vi "CC Main.vi"() -> ()   [LabVIEW 2021]
uses:
  typedefs/CC enum Dither Selection.ctl
  typedefs/CC cluster Hardware Config.ctl
  typedefs/CC cluster Device Index.ctl
  Subsystems/SS cluster Command Queues.ctl
  Subsystems/SS typedef Cmd Queue Reference.ctl
  Subsystems/SS typedef cluster Instrument Command Queue Data.ctl
  hk-channel-class/HK Table/HK Table.lvclass
  typedefs/CC cluster System Settings.ctl
  Subsystems/SS cluster Data Queue type.ctl
  Subsystems/Subsystem Class CryoServer/Subsystem CryoServer.lvclass
  C:/Development/prime/Prime-RIMAS/Subsystems/Subsystem Class.lvclass
  Subsystems/Detector/Detector.lvclass
  Subsystems/Subsystem Class Filter Wheel/Subsystem Filter Wheel.lvclass
  Subsystems/Subsystem Class Telescope/Subsystem Telescope.lvclass
  Subsystems/Subsystem Class Focus/Subsystem Class Focus.lvclass
  Subsystems/Subsystem CryoCooler/Subsystem CryoCooler.lvclass
  Subsystems/Subsystem Pressure Monitor/Subsystem Pressure Monitor.lvclass
  Subsystems/SS cluster Script Status Queue.ctl
  typedefs/CC cluster Observation.ctl
  Observation Queue/CC enum Observation Status.ctl
  Telescope/CC cluster Telescope Offsets.ctl
  typedefs/CC cluster Observation Dither Options.ctl
  library/Activity Log/Activity Log enum Action .ctl
  Subsystems/Subsystem Class.lvclass/Subsystem Class.ctl
  typedefs/CC cluster Script.ctl
  typedefs/CC Script Step.ctl
  typedefs/CC enum Script Action.ctl
  Scripts/CC Rd Wr Script Action.ctl
  typedefs/CC enum Alarm Action.ctl
  Logging/CC enum Current Values Action.ctl
  typedefs/CC cluster Script Status Data.ctl
  Subsystems/SS Read cmd q.vi
  54ac6f3e-f790-48ea-ae38-f3b11f920432.vi
  <vilib>/Utility/TDMS File Viewer/TDMS - File Viewer (NXG Style).vi
  <vilib>/Comparison/Less/Less Functor/Less Functor.lvclass
  <vilib>/regexp/Match Regular Expression.xnode
  Subsystems/Subsystem Class.lvclass
  hk-channel-class/HK Item/HK Item.lvclass
  <vilib>/Utility/TDMS File Viewer/NI_TDMS File Viewer.lvlib
panel:
  in  "Tab Control":T1(tab)
  in  "Priority":i32
  in  "Comment":string
  out "Observation File":string
  in  "Block ID":string
  in  "Images":i32=1 min=1 step=1
  in  "Phase":dbl format="%.1g"
  in  "ROT Offset":dbl
  in  "DECoffset":dbl
  in  "RAoffset":dbl
  in  "Obj Type":string
  in  "Obj Name":string
  in  "Observer":string
  in  "Add to Q top":bool
  in  "Add to Q":bool
  out "Current DEC":string
  out "Current RA":string
  in  "Replace":bool
  in  "Add Obs Row":bool
  in  "Generate Script":bool
  in  "Save Obs List":bool
  in  "Load Obs List":bool
  in  "Radius":dbl format="%.1g"
  in  "Int Time":dbl format="%.1g"
  in  "Spots":i32=1 min=1 step=1
  in  "Dither":T2
  in  "Filter 2":u16(ring) items=["Y", "H", "Open", "J"]
  in  "Filter 1":u16(ring) items=["Z", "Open", "Dark", "NB"]
  in  "DEC":string
  in  "RA":string
  in  "Observation List":i32[](listbox)
  in  "Edit FITS Hdr":bool
  in  "Log 2":bool caption="Log"
  in  "Log":bool
  in  "Export Cryo Data":bool
  out "XY Graph":cluster{timestamp[], dbl[]}[](graph)
  in  "Plot":bool
  in  "Channels":i32[](listbox)
  in  "Open Log":bool
  in  "Note for Log":string
  in  "Send":bool
  in  "Close":bool
  in  "Recent Images":i32(listbox)
  out "Status":string
  out "Progress":u8(slide) scale=0.0..100.0
  out "Current File":string
  in  "Data Folder":path
  out "Temp":bool
  out "Cryo Alarm":bool
  out "Pressure Alarm":bool
  out "Telescope Alarm":bool
  out "FW Alarm":bool
  out "Detector Alarm":bool
  out "Alarm Message":string
  out "Alarm Status":bool
  out "Thumbnail":sgl[][](graph)
  out "Zoom":sgl[][](graph)
  out "Console":string
  out "Waveform Graph":cluster{"image":sgl[]}[](graph)
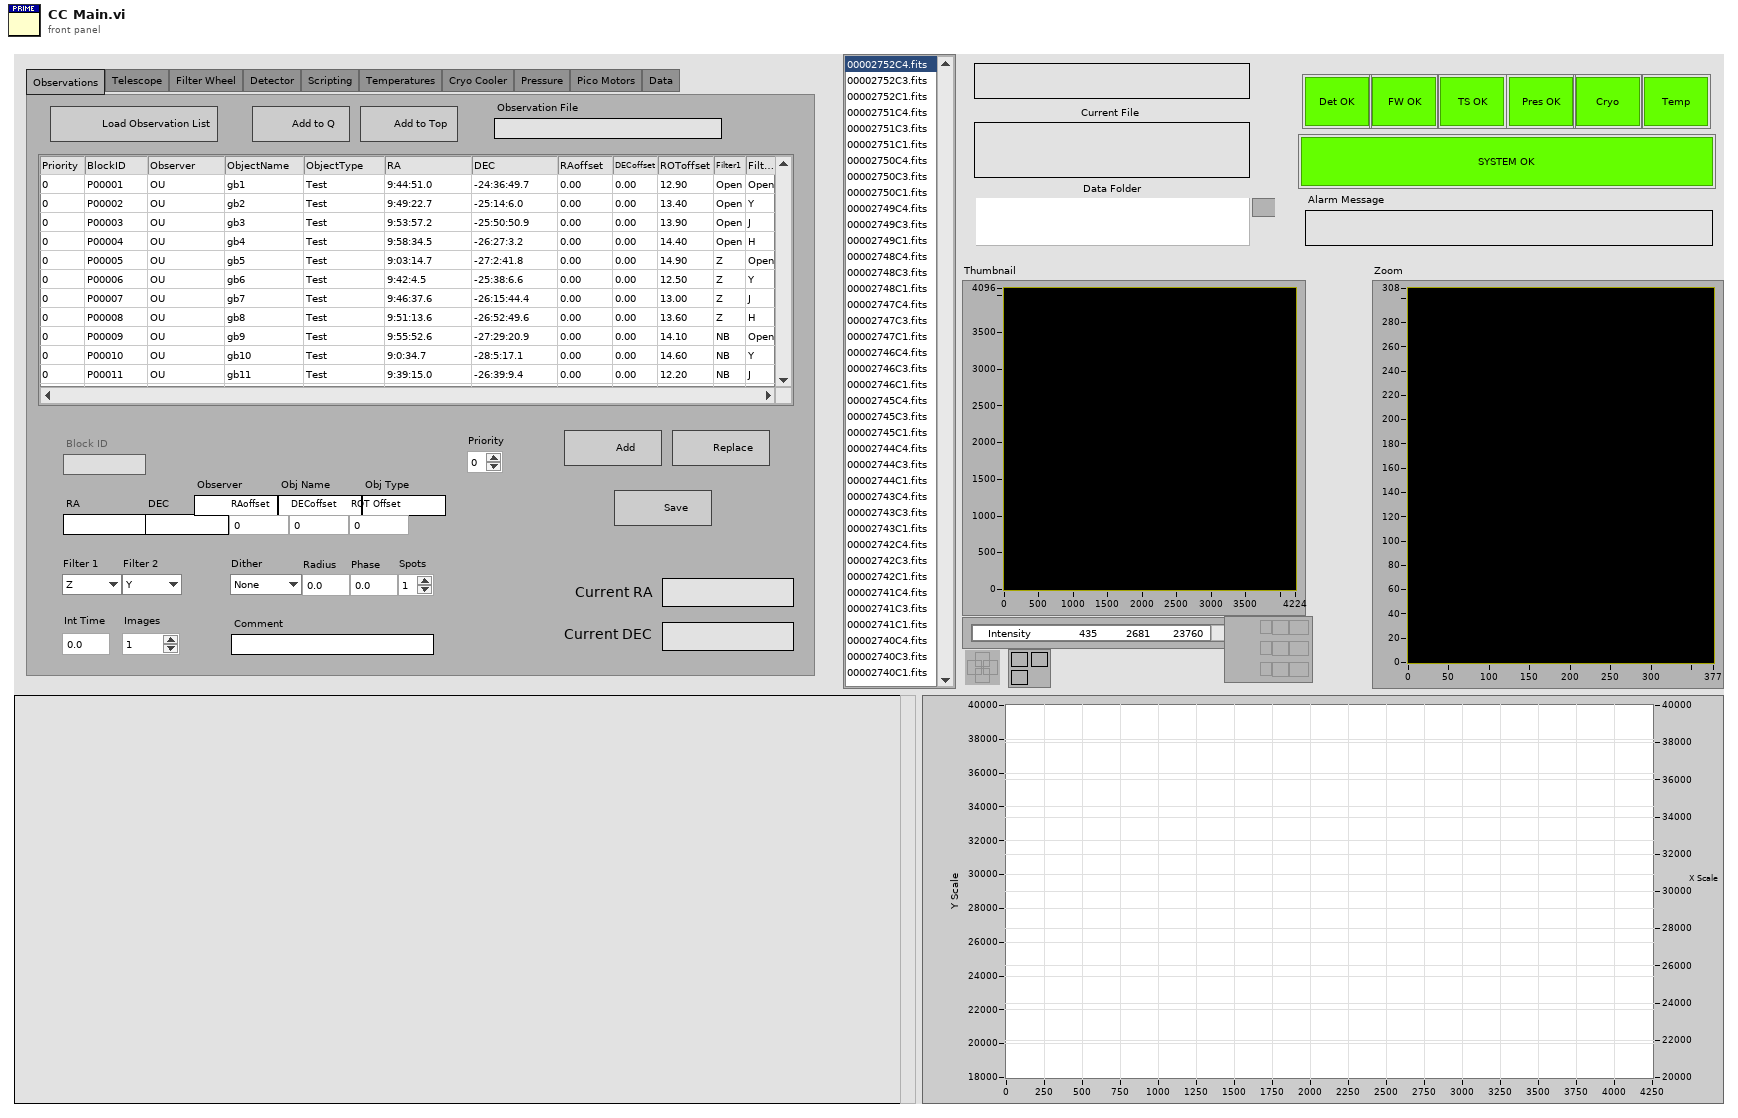
[diagram p1: front panel]
types:
  T1 = enum32{"Observations", "Telescope", "Filter Wheel", "Detector", "Scripting", "Temperatures", "Cryo Cooler", "Pressure", "Pico Motors", "Data"}
  T2 = typedef "CC enum Dither Selection.ctl" = enum16{"None", "Circle", "Random"}
  T3 = enum32{"invalid app kind", "Development System", "Run Time System", "Student Edition", "Embedded LabVIEW", "Evaluation", "Custom"}
  T4 = typedef "CC cluster Hardware Config.ctl" = cluster{"Installed Hardware":T5[]}
  T5 = typedef "CC cluster Device Index.ctl" = cluster{"Device Type Name":string, "Curr Device Name":string, "All Instances":string[]}
  T6 = typedef "SS cluster Command Queues.ctl" = cluster{"Telescope Q":T7, "Filter Wheel Q":T7, "Script Q":T7, "CryoServer Q":T7, "Detector Q":T7, "Focus Q":T7}
  T7 = typedef "SS typedef Cmd Queue Reference.ctl" = refnum<queue>
  T8 = typedef "CC cluster System Settings.ctl" = cluster{"HK Table Name":string, "Images Folder":path, "Obs File":path}
  T9 = typedef "CC cluster Observation.ctl" = cluster{"Priority":i32, "ID":string, "Observer":string, "Obj Name":string, "Obj Type":string, "RA and DEC String":cluster{"RA":string, "DEC":string}, "Filter Wheel 1":string, "Filter Wheel 2":string, "Integration Time":dbl, "Observation Status":T10, "Offsets":T11, "Images":i32, "Dither Options":T12, "Comment 1":string, "Comment 2":string}
  T10 = typedef "CC enum Observation Status.ctl" = enum16{"Ready", "Running", "Done", "Error"}
  T11 = typedef "CC cluster Telescope Offsets.ctl" = cluster{"RA":dbl, "DEC":dbl, "ROT":dbl}
  T12 = typedef "CC cluster Observation Dither Options.ctl" = cluster{"Dither":T2, "Dither Radius":dbl, "Dither Points":i32, "Dither Phase":dbl}
  T13 = cluster{"state":refnum<user-event>, "Hardware":T4, "error":errorcluster, "Cmd Qs":T6, "HK Channels":refnum<class "HK Table.lvclass">, "System Settings":T8, "Data Q":refnum<queue>, "file path":path, "SS":cluster{"CryoServer":refnum<class "Subsystem CryoServer.lvclass">, "Detector":refnum<class "Detector.lvclass">, "Filter Wheel":refnum<class "Subsystem Filter Wheel.lvclass">, "Telescope":refnum<class "Subsystem Telescope.lvclass">, "Focus":refnum<class "Subsystem Class Focus.lvclass">, "CryoCooler":refnum<class "Subsystem CryoCooler.lvclass">, "Pressure":refnum<class "Subsystem Pressure Monitor.lvclass">}, "Script Status Q":refnum<queue>, "Status Data":variant, "curr image":path, "image":sgl[][], "Application:Kind":enum32{"invalid app kind", "Development System", "Run Time System", "Student Edition", "Embedded LabVIEW", "Evaluation", "Custom"}, "Observation List":T9[], "Viewer Ref":refnum<vi>, "Quad Viewer Ref":refnum<vi>, "Obs Queue":refnum<queue>, "Queue vi ref":refnum<vi>, "Script Running":bool}
  T14 = typedef "SS cluster Data Queue type.ctl" = cluster{"Source":string, "Type":string, "Data":variant}
  T15 = typedef "Activity Log enum Action .ctl" = enum16{"Add Entry", "Get Log", "Restore From Disk", "Save to Disk", "Init"}
  T16 = typedef "SS typedef cluster Instrument Command Queue Data.ctl" = cluster{"Cmd":string, "Parameters":variant}
  T17 = typedef "CC Rd Wr Script Action.ctl" = enum16{"Read", "Write", "List", "Delete"}
  T18 = typedef "CC cluster Script.ctl" = cluster{"Name":string, "Script":T19[]}
  T19 = typedef "CC Script Step.ctl" = cluster{"Action":T20, "Data":variant}
  T20 = typedef "CC enum Script Action.ctl" = enum16{"Noop", "Define Object", "Define Exposure", "Define Dithering", "Acquire Images", "Set Filter Wheel", "Telescope Home", "Telescope Move", "Telescope RA DEC", "Focus Move Relative", "Focus Move Absolute", "Focus Set Home", "Macro", "Pause", "Ask User", "Define Random Dither"}
  T21 = typedef "CC enum Alarm Action.ctl" = enum16{"Init", "Add Alarm", "Get Alarms", "Clear Alarm", "Clear All Alarms"}
  T22 = typedef "CC enum Current Values Action.ctl" = enum16{"Init", "Write Item", "Write Array", "Read Item", "Read Array", "Read All", "Add Channels", "New File", "Add Message", "Get Current Values", "Close"}
  T23 = typedef "CC cluster Script Status Data.ctl" = cluster{"Time":timestamp, "Running":bool, "Step":i32, "Script Name":string, "Step Name":string}
  T24 = typedef "SS cluster Script Status Queue.ctl" = cluster{"Msg":string, "Data":variant}
  T25 = enum8{"Enabled", "Disabled", "Disabled and Grayed Out"}
  T26 = typedef "CC cluster Script Panel Defaults.ctl" = cluster{"Script Name":string, "Script Path":path}
  T27 = typedef "CC cluster Alarm Data.ctl" = cluster{"Measured Value":dbl, "Alarm Low":dbl, "Alarm High":dbl, "Message":string, "Source":string}
  T28 = typedef "LVRectTypeDef.ctl" = cluster{"Left":i16, "Top":i16, "Right":i16, "Bottom":i16}
  T29 = cluster{"CryoServer":refnum<class "Subsystem CryoServer.lvclass">, "Detector":refnum<class "Detector.lvclass">, "Filter Wheel":refnum<class "Subsystem Filter Wheel.lvclass">, "Telescope":refnum<class "Subsystem Telescope.lvclass">, "Focus":refnum<class "Subsystem Class Focus.lvclass">, "CryoCooler":refnum<class "Subsystem CryoCooler.lvclass">, "Pressure":refnum<class "Subsystem Pressure Monitor.lvclass">}
  T30 = typedef "LVPoint32TypeDef.ctl" = cluster{"Horizontal":i32, "Vertical":i32}
  T31 = typedef "LVRowAndColumnTypeDef.ctl" = cluster{"Row":i32, "Column":i32}
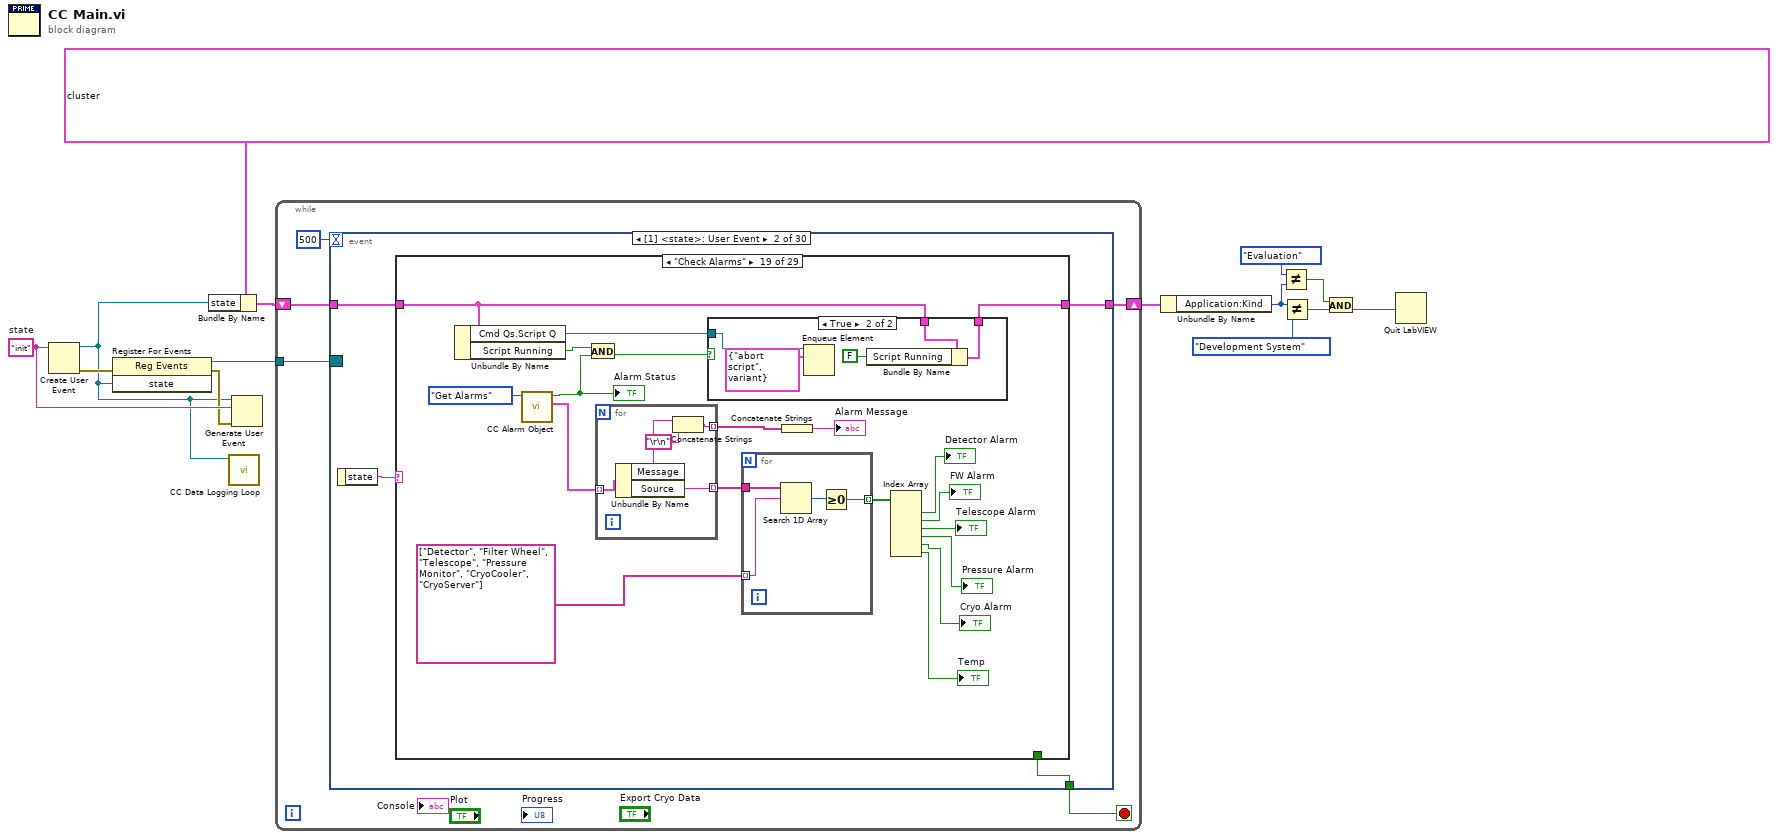
[diagram p0: block diagram]
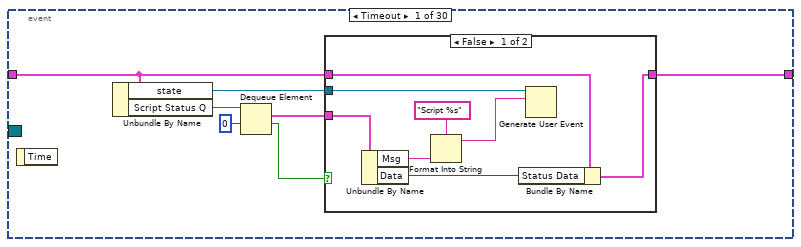
[diagram p2: hidden frame]
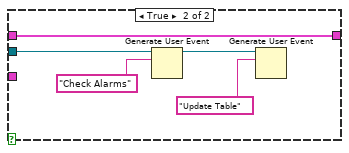
[diagram p3: hidden frame]
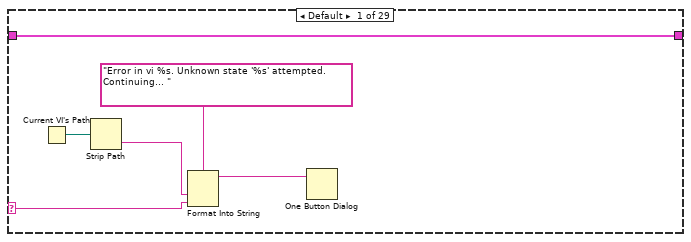
[diagram p4: hidden frame]
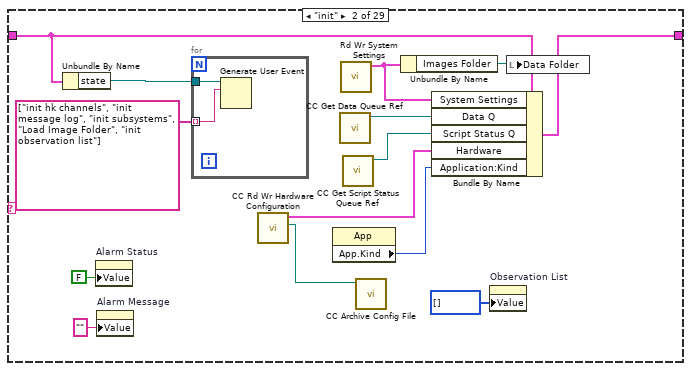
[diagram p5: hidden frame]
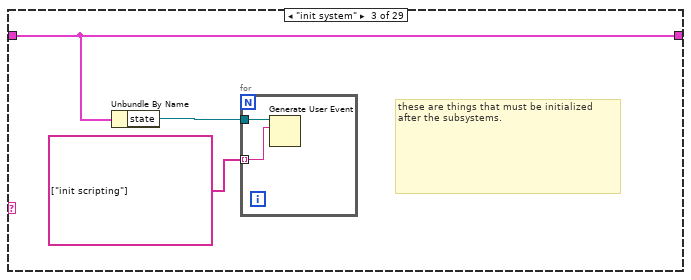
[diagram p6: hidden frame]
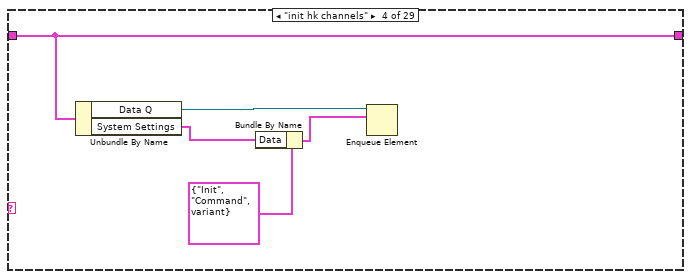
[diagram p7: hidden frame]
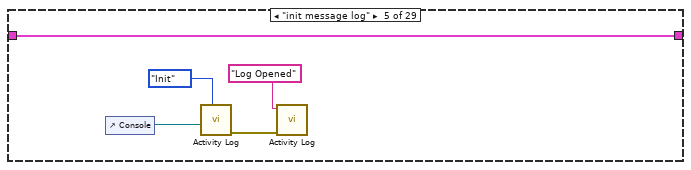
[diagram p8: hidden frame]
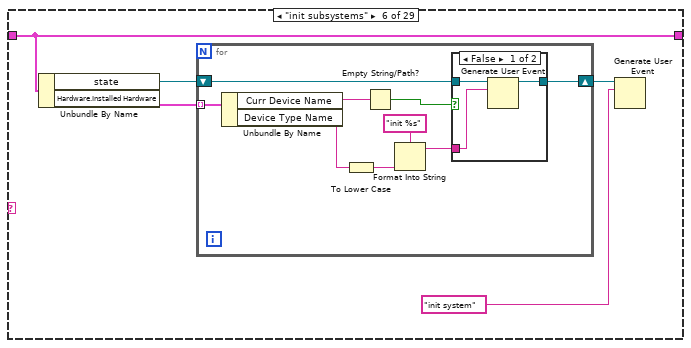
[diagram p9: hidden frame]
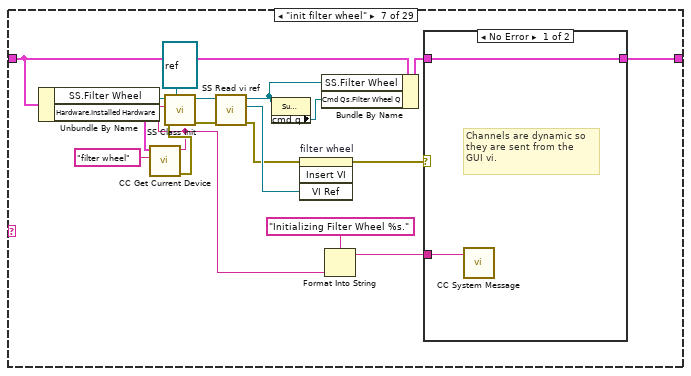
[diagram p11: hidden frame]
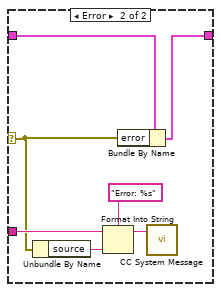
[diagram p12: hidden frame]
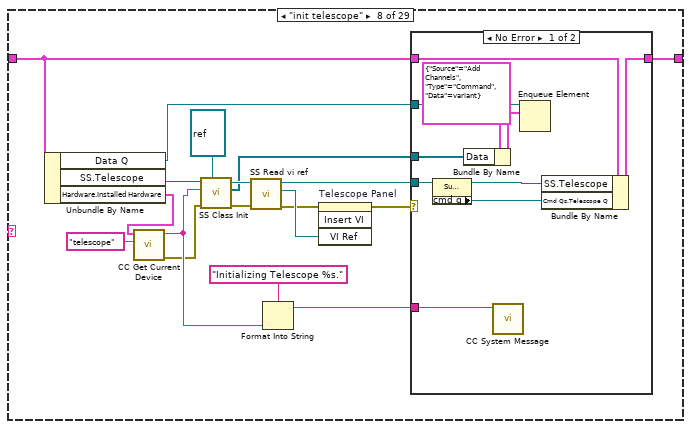
[diagram p13: hidden frame]
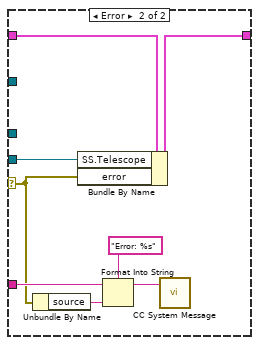
[diagram p14: hidden frame]
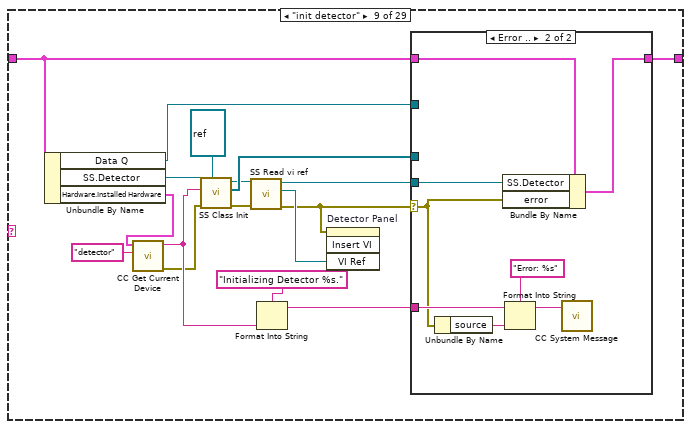
[diagram p15: hidden frame]
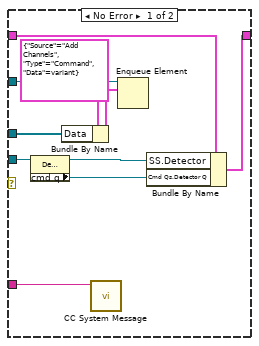
[diagram p16: hidden frame]
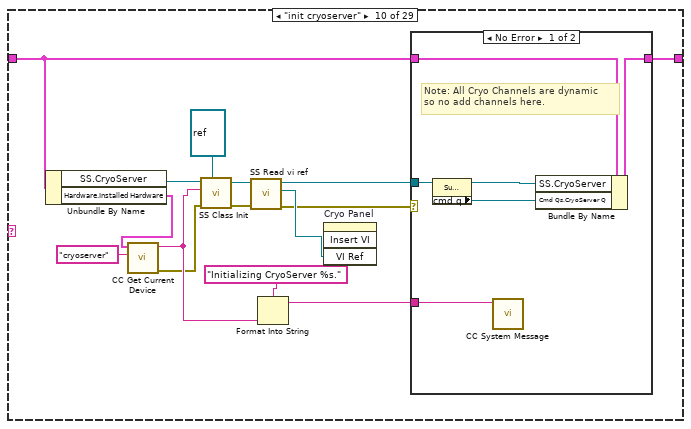
[diagram p17: hidden frame]
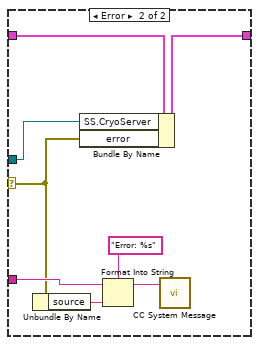
[diagram p18: hidden frame]
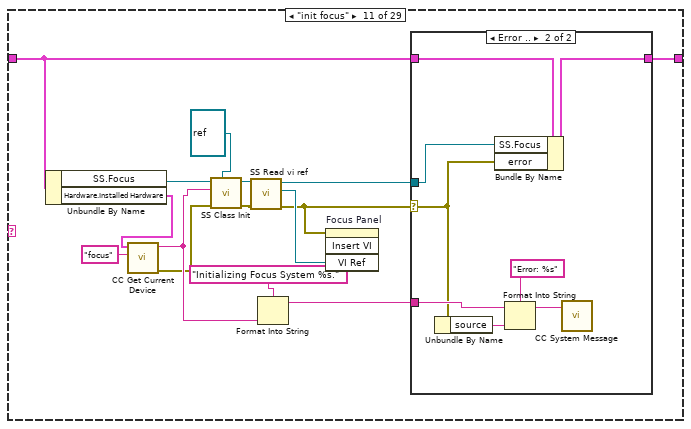
[diagram p19: hidden frame]
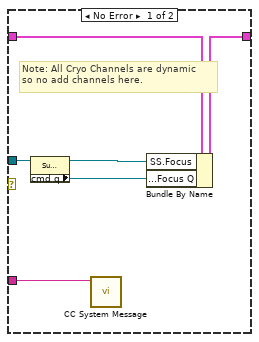
[diagram p20: hidden frame]
diagram:
  w11 = "init"  # state
  n1 = Create User Event(user event datatype=w11) -> (user event=w8:refnum<user-event>, error out=w9:errorcluster)  [unwired: 1 in]
  n2 = register-events(error in=w9, w8) -> (reference out=w12:refnum<event-registration>, error out=w10:errorcluster)  [unwired: 1 in]
  n3 = Bundle By Name(cluster=T13 {"state"=refnum, "Hardware"={"Installed Hardware"=[]}, "error"={"status"=FALSE, "code"=0, "source"=""}, "Cmd Qs"={"Telescope Q"=refnum, "Filter Wheel Q"=refnum, "Script Q"=refnum, "CryoServer Q"=refnum, "Detector Q"=refnum, "Focus Q"=refnum}, "HK Channels"=refnum, "System Settings"={"HK Table Name"="", "Images Folder"=path "", "Obs File"=path ""}, "Data Q"=refnum, "file path"=path "", "SS"={"CryoServer"=refnum, "Detector"=refnum, "Filter Wheel"=refnum, "Telescope"=refnum, "Focus"=refnum, "CryoCooler"=refnum, "Pressure"=refnum}, "Script Status Q"=refnum, "Status Data"=variant, "curr image"=path "", "image"=[], "Application:Kind"=enum."invalid app kind", "Observation List"=[], "Viewer Ref"=refnum, "Quad Viewer Ref"=refnum, "Obs Queue"=refnum, "Queue vi ref"=refnum, "Script Running"=FALSE}, "state"=w8) -> (w13:T13)
  n4 = call "CC Data Logging Loop.vi"("user event"=w8) -> ()  [unwired: 11 in]
  n5 = Generate User Event(user event=w8, event data cluster=w11, error in=w10) -> ()  [unwired: 1 in, 2 out]
  n6 = while {
    tunnel: w12 -> [w19]
    shift-right: [w17] -> w7
    shift-left: w13 -> [w18]
    stop <- w16 stop-if-true
    n7 = event shown="[1] <state>: User Event" {
      selector: w19 -> [_ _ _ _ _ _ _ _ _ _ _ _ _ _ _ _ _ _ _ _ _ _ _ _ _ _ _ _ _ _]
      dyn-events: _ -> [_ _ _ _ _ _ _ _ _ _ _ _ _ _ _ _ _ _ _ _ _ _ _ _ _ _ _ _ _ _]
      timeout: 500 -> [_ _ _ _ _ _ _ _ _ _ _ _ _ _ _ _ _ _ _ _ _ _ _ _ _ _ _ _ _ _]
      tunnel: w18 -> [w24 w42 w589 w654 w656 w659 w677 w708 w717 w726 w759 w793 w799 w804 w810 w816 w819 w821 w828 w966 w979 w996 w999 w1002 w1004 w1008 w1009 w1017 w1031 w1037]
      tunnel: [w21 w41 w588 w654 w656 w661 w677 w708 w714 w727 w760 w793 w799 w804 w810 w816 w819 w821 w829 w966 w981 w996 w999 w1002 w1004 w1008 w1009 w1013 w1031 w1034] -> w17
      tunnel: [_ w40 _ _ _ _ _ _ _ _ _ _ _ _ _ _ _ _ _ _ _ _ _ _ _ FALSE ("Close") _ _ _ _] -> w16
      event Timeout {
        n8 = event-data() -> ()  [unwired: 1 in, 1 out]
        n9 = Unbundle By Name(w24) -> ("state"=w23:refnum<user-event>, "Script Status Q"=w26:refnum<queue>)
        n10 = Dequeue Element(queue=w26, timeout in ms (-1)=0) -> (element=w22:T24, timed out?=w25:bool)  [unwired: 1 in, 2 out]
        n11 = case shown="False" w25 {
          tunnel: w24 -> [w29 w39]
          tunnel: w23 -> [w34 w38]
          tunnel: w22 -> [w33 _]
          tunnel: [w27 w39] -> w21
          frame False {
            n12 = Unbundle By Name(w33) -> ("Msg"=w31:string, "Data"=w28:variant)
            n13 = Format Into String(format string="Script %s", w31) -> (resulting string=w30:string)  [unwired: 2 in, 1 out]
            n14 = Bundle By Name(cluster=w29, "Status Data"=w28) -> (w27:T13)
            n15 = Generate User Event(user event=w34, event data cluster=w30) -> ()  [unwired: 2 in, 2 out]
          }
          frame True {
            n16 = Generate User Event(user event=w38, event data cluster="Check Alarms" ("event data")) -> (user event out=w36:refnum<user-event>)  [unwired: 2 in, 1 out]
            n17 = Generate User Event(user event=w36, event data cluster="Update Table" ("event data")) -> ()  [unwired: 2 in, 2 out]
          }
        }
      }
      event User Event {
        n18 = event-data() -> ("state"=w43:string)  [unwired: 1 in]
        n19 = case shown="\"Check Alarms\"" w43 {
          selector: w43 -> [w48 _ _ _ _ _ _ _ _ _ _ _ _ _ _ _ _ _ _ _ _ _ _ _ _ _ _ _ _]
          tunnel: w42 -> [w44 w60 w67 w71 w80 w85 w109 w139 w176 w207 w239 w270 w305 w327 w356 w375 w382 w385 w403 w448 w474 w504 w518 w524 w531 w551 w559 w568 w578]
          tunnel: [w44 w61 w67 w71 w80 w85 w110 w140 w177 w208 w240 w271 w306 w328 w357 w375 w382 w385 w404 w448 w474 w505 w518 w524 w532 w551 w559 w568 w578] -> w41
          tunnel: [_ _ _ _ _ _ _ _ _ _ _ _ _ _ _ _ _ _ _ _ _ _ _ _ _ _ _ FALSE TRUE] -> w40
          frame Default {
            n20 = Current VI's Path() -> (path=w47:path)
            n21 = Strip Path(path=w47) -> (name=w46:string)  [unwired: 1 out]
            n22 = Format Into String(format string="Error in vi %s. Unknown state '%s' attempted. Continuing... ", w46, w48) -> (resulting string=w45:string)  [unwired: 2 in, 1 out]
            n23 = One Button Dialog(message=w45) -> ()  [unwired: 1 in, 1 out]
          }
          frame "init" {
            n24 = Unbundle By Name(w60) -> ("state"=w63:refnum<user-event>)
            n25 = property on="Alarm Status" class="Bool (strict)"("Value"=FALSE ("Alarm Status")) -> ()  [unwired: 2 in, 2 out]
            n26 = property on="Alarm Message" class="Str"("Value"="" ("Alarm Message")) -> ()  [unwired: 2 in, 2 out]
            n27 = for {
              tunnel: w63 -> [w65]
              tunnel: string[] ["init hk channels", "init message log", "init subsystems", "Load Image Folder", "init observation list"] -> [w64] mode=indexing
              n28 = Generate User Event(user event=w65, event data cluster=w64) -> ()  [unwired: 2 in, 2 out]
            }
            n29 = call "CC Rd Wr Hardware Configuration.vi"() -> ("File"=w54:path, "Hardware Config out"=w55:T4)  [unwired: 9 in, 1 out]
            n30 = property class="App"() -> ("App.Kind"=w53:T3)  [unwired: 2 in, 2 out]
            n31 = call "CC Get Data Queue Ref.vi"() -> ("Data Q"=w59:refnum<queue>)  [unwired: 10 in, 1 out]
            n32 = call "Rd Wr System Settings.vi"() -> ("System Settings out"=w57:T8)  [unwired: 10 in, 1 out]
            n33 = call "CC Get Script Status Queue Ref.vi"() -> ("Script Status Q"=w58:refnum<queue>)  [unwired: 10 in, 1 out]
            n34 = call "CC Archive Config File.vi"("config file"=w54) -> ()  [unwired: 10 in, 1 out]
            n35 = Unbundle By Name(w57) -> ("Images Folder"=w56:path)
            n36 = Bundle By Name(cluster=w60, "System Settings"=w57, "Data Q"=w59, "Script Status Q"=w58, "Hardware"=w55, "Application:Kind"=w53) -> (w61:T13)
            n37 = property on="Observation List" class="MCListbox (strict)"("Value"=i32[] [] ("Observation List")) -> ()  [unwired: 2 in, 2 out]
            n38 = local write "Data Folder"(w56) -> ()
          }
          frame "init system" {
            # "these are things that must be initialized after the subsystems."
            n39 = Unbundle By Name(w67) -> ("state"=w68:refnum<user-event>)
            n40 = for {
              tunnel: w68 -> [w70]
              tunnel: string[] ["init scripting"] -> [w69] mode=indexing
              n41 = Generate User Event(user event=w70, event data cluster=w69) -> ()  [unwired: 2 in, 2 out]
            }
          }
          frame "init hk channels" {
            n42 = Unbundle By Name(w71) -> ("Data Q"=w75:refnum<queue>, "System Settings"=w73:T8)
            n43 = Bundle By Name(cluster=T14 {"Source"="Init", "Type"="Command", "Data"=variant} ("element"), "Data"=w73) -> (w72:T14)
            n44 = Enqueue Element(queue=w75, element=w72) -> ()  [unwired: 2 in, 3 out]
          }
          frame "init message log" {
            n45 = control-ref of="Console"() -> (w78:refnum<vi>)
            n46 = call "Activity Log.vi"("Action"=Activity_Log_enum_Action_."Init", "string ref"=w78) -> ("Error Out"=w77:errorcluster)  [unwired: 8 in, 1 out]
            n47 = call "Activity Log.vi"("Error In"=w77, "Message Log Entry"="Log Opened") -> ()  [unwired: 8 in, 2 out]
          }
          frame "init subsystems" {
            n48 = Unbundle By Name(w85) -> ("state"=w84:refnum<user-event>, "Hardware.Installed Hardware"=w83:T5[])
            n49 = for {
              tunnel: w83 -> [w92] mode=indexing
              shift-right: [w86] -> w82
              shift-left: w84 -> [w93]
              n50 = Unbundle By Name(w92) -> ("Curr Device Name"=w88:string, "Device Type Name"=w87:string)
              n51 = To Lower Case(string=w87) -> (all lower case string=w89:string)
              n52 = Empty String/Path?(string/path=w88) -> (empty?=w94:bool)
              n53 = Format Into String(format string="init %s", w89) -> (resulting string=w91:string)  [unwired: 2 in, 1 out]
              n54 = case shown="False" w94 {
                tunnel: w93 -> [w97 w98]
                tunnel: w91 -> [w96 _]
                tunnel: [w95 w98] -> w86
                frame False {
                  n55 = Generate User Event(user event=w97, event data cluster=w96) -> (user event out=w95:refnum<user-event>)  [unwired: 2 in, 1 out]
                }
                frame True {
                }
              }
            }
            n56 = Generate User Event(user event=w82, event data cluster="init system" ("format string")) -> ()  [unwired: 2 in, 2 out]
          }
          frame "init filter wheel" {
            n57 = Unbundle By Name(w109) -> ("SS.Filter Wheel"=w108:refnum<class "Subsystem Filter Wheel.lvclass">, "Hardware.Installed Hardware"=w102:T5[])
            n58 = call "CC Get Current Device.vi"("Device Type Name"="filter wheel", "Hardware.Installed Hardware"=w102) -> ("error out"=w100:errorcluster, "Curr Device Name"=w99:string)  [unwired: 7 in, 1 out]
            n59 = call-dynamic "SS Class Init.vi"("VI Refnum"=refnum<vi> refnum, "error in (no error)"=w100, "Device"=w99, "Subsystem Filter Wheel in"=w108) -> ("error out"=w104:errorcluster, "Subsystem Filter Wheel out"=w107:refnum<class "Subsystem Filter Wheel.lvclass">)  [unwired: 5 in, 1 out]
            n60 = call "SS Read vi ref.vi"("error in (no error)"=w104, "Subsystem Class in"=w107) -> ("error out"=w115:errorcluster, "vi ref"=w116:refnum<vi>, "Subsystem Class out"=w106:refnum<class "Subsystem Filter Wheel.lvclass">)  [unwired: 7 in]
            n61 = property class="Subsystem Filter Wheel.lvclass"(reference=w106) -> ("cmd q"=w105:T7)  [unwired: 1 in, 2 out]
            n62 = invoke on="filter wheel" class="SubPnl" method="Insert VI"(error in=w115, "VI Ref"=w116) -> (error out=w113:errorcluster)  [unwired: 2 in, 3 out]
            n63 = Bundle By Name(cluster=w109, "SS.Filter Wheel"=w106, "Cmd Qs.Filter Wheel Q"=w105) -> (w111:T13)
            n64 = Format Into String(format string="Initializing Filter Wheel %s.", w99) -> (resulting string=w112:string)  [unwired: 2 in, 1 out]
            n65 = case shown="No Error" w113 {
              selector: w113 -> [_ w121]
              tunnel: w112 -> [w118 w122]
              tunnel: w111 -> [w117 w125]
              tunnel: [w117 w124] -> w110
              frame No Error {
                # "Channels are dynamic so\nthey are sent from the \nGUI vi."
                n66 = call "CC System Message.vi"("Message"=w118) -> ()  [unwired: 10 in, 1 out]
              }
              frame Error {
                n67 = Unbundle By Name(w121) -> ("source"=w120:string)
                n68 = Format Into String(format string="Error: %s", initial string=w122, w120) -> (resulting string=w119:string)  [unwired: 1 in, 1 out]
                n69 = Bundle By Name(cluster=w125, "error"=w121) -> (w124:T13)
                n70 = call "CC System Message.vi"("Message"=w119) -> ()  [unwired: 10 in, 1 out]
              }
            }
          }
          frame "init telescope" {
            n71 = Unbundle By Name(w139) -> ("Data Q"=w131:refnum<queue>, "SS.Telescope"=w143:refnum<class "Subsystem Telescope.lvclass">, "Hardware.Installed Hardware"=w128:T5[])
            n72 = call "CC Get Current Device.vi"("Device Type Name"="telescope", "Hardware.Installed Hardware"=w128) -> ("error out"=w126:errorcluster, "Curr Device Name"=w127:string)  [unwired: 7 in, 1 out]
            n73 = call-dynamic "SS Class Init.vi"("VI Refnum"=refnum<vi> refnum, "error in (no error)"=w126, "Device"=w127, "Telescope in"=w143) -> ("error out"=w141:errorcluster, "Channel List"=w132:refnum<class "HK Item.lvclass">[], "Telescope out"=w142:refnum<class "Subsystem Telescope.lvclass">)  [unwired: 5 in]
            n74 = call "SS Read vi ref.vi"("error in (no error)"=w141, "Subsystem Class in"=w142) -> ("error out"=w134:errorcluster, "vi ref"=w135:refnum<vi>, "Subsystem Class out"=w136:refnum<class "Subsystem Telescope.lvclass">)  [unwired: 7 in]
            n75 = Format Into String(format string="Initializing Telescope %s.", w127) -> (resulting string=w137:string)  [unwired: 2 in, 1 out]
            n76 = invoke on="Telescope Panel" class="SubPnl" method="Insert VI"(error in=w134, "VI Ref"=w135) -> (error out=w133:errorcluster)  [unwired: 2 in, 3 out]
            n77 = case shown="No Error" w133 {
              selector: w133 -> [_ w157]
              tunnel: w137 -> [w144 w158]
              tunnel: w139 -> [w150 w161]
              tunnel: [w151 w160] -> w140
              tunnel: w136 -> [w153 w155]
              tunnel: w132 -> [w146 _]
              tunnel: w131 -> [w148 _]
              frame No Error {
                n78 = property class="Subsystem Telescope.lvclass"(reference=w153) -> (reference out=w149:refnum<class "Subsystem Telescope.lvclass">, "cmd q"=w152:T7)  [unwired: 1 in, 1 out]
                n79 = Bundle By Name(cluster=T14 {"Source"="Add Channels", "Type"="Command", "Data"=variant} ("element"), "Data"=w146) -> (w145:T14)
                n80 = call "CC System Message.vi"("Message"=w144) -> ()  [unwired: 10 in, 1 out]
                n81 = Enqueue Element(queue=w148, element=w145) -> ()  [unwired: 2 in, 3 out]
                n82 = Bundle By Name(cluster=w150, "SS.Telescope"=w149, "Cmd Qs.Telescope Q"=w152) -> (w151:T13)
              }
              frame Error {
                n83 = Unbundle By Name(w157) -> ("source"=w156:string)
                n84 = Bundle By Name(cluster=w161, "SS.Telescope"=w155, "error"=w157) -> (w160:T13)
                n85 = Format Into String(format string="Error: %s", initial string=w158, w156) -> (resulting string=w154:string)  [unwired: 1 in, 1 out]
                n86 = call "CC System Message.vi"("Message"=w154) -> ()  [unwired: 10 in, 1 out]
              }
            }
          }
          frame "init detector" {
            n87 = Unbundle By Name(w176) -> ("Data Q"=w171:refnum<queue>, "SS.Detector"=w169:refnum<class "Detector.lvclass">, "Hardware.Installed Hardware"=w166:T5[])
            n88 = call "CC Get Current Device.vi"("Device Type Name"="detector", "Hardware.Installed Hardware"=w166) -> ("error out"=w164:errorcluster, "Curr Device Name"=w165:string)  [unwired: 7 in, 1 out]
            n89 = call-dynamic "SS Class Init.vi"("VI Refnum"=refnum<vi> refnum, "error in (no error)"=w164, "Device"=w165, "Detector in"=w169) -> ("error out"=w178:errorcluster, "Channel List"=w172:refnum<class "HK Item.lvclass">[], "Detector out"=w168:refnum<class "Detector.lvclass">)  [unwired: 5 in]
            n90 = call "SS Read vi ref.vi"("error in (no error)"=w178, "Subsystem Class in"=w168) -> ("error out"=w162:errorcluster, "vi ref"=w163:refnum<vi>, "Subsystem Class out"=w173:refnum<class "Detector.lvclass">)  [unwired: 7 in]
            n91 = Format Into String(format string="Initializing Detector %s.", w165) -> (resulting string=w174:string)  [unwired: 2 in, 1 out]
            n92 = invoke on="Detector Panel" class="SubPnl" method="Insert VI"(error in=w162, "VI Ref"=w163) -> ()  [unwired: 2 in, 4 out]
            n93 = case shown="Error .." w162 {
              selector: w162 -> [_ w192]
              tunnel: w174 -> [w179 w193]
              tunnel: w176 -> [w185 w196]
              tunnel: [w186 w195] -> w177
              tunnel: w173 -> [w188 w190]
              tunnel: w172 -> [w181 _]
              tunnel: w171 -> [w183 _]
              frame No Error {
                n94 = property class="Detector.lvclass"(reference=w188) -> (reference out=w184:refnum<class "Detector.lvclass">, "cmd q"=w187:T7)  [unwired: 1 in, 1 out]
                n95 = Bundle By Name(cluster=T14 {"Source"="Add Channels", "Type"="Command", "Data"=variant} ("element"), "Data"=w181) -> (w180:T14)
                n96 = call "CC System Message.vi"("Message"=w179) -> ()  [unwired: 10 in, 1 out]
                n97 = Enqueue Element(queue=w183, element=w180) -> ()  [unwired: 2 in, 3 out]
                n98 = Bundle By Name(cluster=w185, "SS.Detector"=w184, "Cmd Qs.Detector Q"=w187) -> (w186:T13)
              }
              frame Error {
                n99 = Unbundle By Name(w192) -> ("source"=w191:string)
                n100 = Bundle By Name(cluster=w196, "SS.Detector"=w190, "error"=w192) -> (w195:T13)
                n101 = Format Into String(format string="Error: %s", initial string=w193, w191) -> (resulting string=w189:string)  [unwired: 1 in, 1 out]
                n102 = call "CC System Message.vi"("Message"=w189) -> ()  [unwired: 10 in, 1 out]
              }
            }
          }
          frame "init cryoserver" {
            n103 = Unbundle By Name(w207) -> ("SS.CryoServer"=w211:refnum<class "Subsystem CryoServer.lvclass">, "Hardware.Installed Hardware"=w200:T5[])
            n104 = call "CC Get Current Device.vi"("Device Type Name"="cryoserver", "Hardware.Installed Hardware"=w200) -> ("error out"=w198:errorcluster, "Curr Device Name"=w199:string)  [unwired: 7 in, 1 out]
            n105 = call-dynamic "SS Class Init.vi"("VI Refnum"=refnum<vi> refnum, "error in (no error)"=w198, "Device"=w199, "Subsystem CryoServer in"=w211) -> ("error out"=w209:errorcluster, "Subsystem CryoServer out"=w210:refnum<class "Subsystem CryoServer.lvclass">)  [unwired: 5 in, 1 out]
            n106 = call "SS Read vi ref.vi"("error in (no error)"=w209, "Subsystem Class in"=w210) -> ("error out"=w197:errorcluster, "vi ref"=w202:refnum<vi>, "Subsystem Class out"=w204:refnum<class "Subsystem CryoServer.lvclass">)  [unwired: 7 in]
            n107 = Format Into String(format string="Initializing CryoServer %s.", w199) -> (resulting string=w205:string)  [unwired: 2 in, 1 out]
            n108 = invoke on="Cryo Panel" class="SubPnl" method="Insert VI"("VI Ref"=w202) -> ()  [unwired: 3 in, 4 out]
            n109 = case shown="No Error" w197 {
              selector: w197 -> [_ w221]
              tunnel: w205 -> [w212 w222]
              tunnel: w207 -> [w214 w225]
              tunnel: [w215 w224] -> w208
              tunnel: w204 -> [w217 w219]
              frame No Error {
                # "Note: All Cryo Channels are dynamic\nso no add channels here."
                n110 = property class="Subsystem CryoServer.lvclass"(reference=w217) -> (reference out=w213:refnum<class "Subsystem CryoServer.lvclass">, "cmd q"=w216:T7)  [unwired: 1 in, 1 out]
                n111 = call "CC System Message.vi"("Message"=w212) -> ()  [unwired: 10 in, 1 out]
                n112 = Bundle By Name(cluster=w214, "SS.CryoServer"=w213, "Cmd Qs.CryoServer Q"=w216) -> (w215:T13)
              }
              frame Error {
                n113 = Unbundle By Name(w221) -> ("source"=w220:string)
                n114 = Bundle By Name(cluster=w225, "SS.CryoServer"=w219, "error"=w221) -> (w224:T13)
                n115 = Format Into String(format string="Error: %s", initial string=w222, w220) -> (resulting string=w218:string)  [unwired: 1 in, 1 out]
                n116 = call "CC System Message.vi"("Message"=w218) -> ()  [unwired: 10 in, 1 out]
              }
            }
          }
          frame "init focus" {
            n117 = Unbundle By Name(w239) -> ("SS.Focus"=w232:refnum<class "Subsystem Class Focus.lvclass">, "Hardware.Installed Hardware"=w234:T5[])
            n118 = call "CC Get Current Device.vi"("Device Type Name"="focus", "Hardware.Installed Hardware"=w234) -> ("error out"=w229:errorcluster, "Curr Device Name"=w230:string)  [unwired: 7 in, 1 out]
            n119 = call-dynamic "SS Class Init.vi"("VI Refnum"=refnum<vi> refnum, "error in (no error)"=w229, "Device"=w230, "Subsystem Class Focus in"=w232) -> ("error out"=w227:errorcluster, "Subsystem Class Focus out"=w228:refnum<class "Subsystem Class Focus.lvclass">)  [unwired: 5 in, 1 out]
            n120 = call "SS Read vi ref.vi"("error in (no error)"=w227, "Subsystem Class in"=w228) -> ("error out"=w226:errorcluster, "vi ref"=w233:refnum<vi>, "Subsystem Class out"=w236:refnum<class "Subsystem Class Focus.lvclass">)  [unwired: 7 in]
            n121 = Format Into String(format string="Initializing Focus System %s.", w230) -> (resulting string=w237:string)  [unwired: 2 in, 1 out]
            n122 = invoke on="Focus Panel" class="SubPnl" method="Insert VI"(error in=w226, "VI Ref"=w233) -> ()  [unwired: 2 in, 4 out]
            n123 = case shown="Error .." w226 {
              selector: w226 -> [_ w250]
              tunnel: w237 -> [w242 w251]
              tunnel: w239 -> [w244 w254]
              tunnel: [w245 w253] -> w240
              tunnel: w236 -> [w246 w248]
              frame No Error {
                # "Note: All Cryo Channels are dynamic\nso no add channels here."
                n124 = property class="Subsystem Class Focus.lvclass"(reference=w246) -> (reference out=w243:refnum<class "Subsystem Class Focus.lvclass">, "cmd q"=w241:T7)  [unwired: 1 in, 1 out]
                n125 = call "CC System Message.vi"("Message"=w242) -> ()  [unwired: 10 in, 1 out]
                n126 = Bundle By Name(cluster=w244, "SS.Focus"=w243, "Cmd Qs.Focus Q"=w241) -> (w245:T13)
              }
              frame Error {
                n127 = Unbundle By Name(w250) -> ("source"=w249:string)
                n128 = Bundle By Name(cluster=w254, "SS.Focus"=w248, "error"=w250) -> (w253:T13)
                n129 = Format Into String(format string="Error: %s", initial string=w251, w249) -> (resulting string=w247:string)  [unwired: 1 in, 1 out]
                n130 = call "CC System Message.vi"("Message"=w247) -> ()  [unwired: 10 in, 1 out]
              }
            }
          }
          frame "init cryocooler" {
            n131 = Unbundle By Name(w270) -> ("Data Q"=w255:refnum<queue>, "SS.CryoCooler"=w264:refnum<class "Subsystem CryoCooler.lvclass">, "Hardware.Installed Hardware"=w265:T5[])
            n132 = call "CC Get Current Device.vi"("Device Type Name"="cryocooler", "Hardware.Installed Hardware"=w265) -> ("error out"=w261:errorcluster, "Curr Device Name"=w262:string)  [unwired: 7 in, 1 out]
            n133 = call-dynamic "SS Class Init.vi"("VI Refnum"=refnum<vi> refnum, "error in (no error)"=w261, "Device"=w262, "Subsystem CryoCooler in"=w264) -> ("error out"=w259:errorcluster, "Channel List"=w256:refnum<class "HK Item.lvclass">[], "Subsystem CryoCooler out"=w260:refnum<class "Subsystem CryoCooler.lvclass">)  [unwired: 5 in]
            n134 = call "SS Read vi ref.vi"("error in (no error)"=w259, "Subsystem Class in"=w260) -> ("error out"=w258:errorcluster, "vi ref"=w257:refnum<vi>, "Subsystem Class out"=w267:refnum<class "Subsystem CryoCooler.lvclass">)  [unwired: 7 in]
            n135 = Format Into String(format string="Initializing CryoCooler System %s.", w262) -> (resulting string=w268:string)  [unwired: 2 in, 1 out]
            n136 = invoke on="Telescope Panel" class="SubPnl" method="Insert VI"("VI Ref"=w257) -> ()  [unwired: 3 in, 4 out]
            n137 = case shown="No Error" w258 {
              selector: w258 -> [_ w285]
              tunnel: w268 -> [w277 w286]
              tunnel: w270 -> [w279 w289]
              tunnel: [w280 w288] -> w271
              tunnel: w267 -> [w281 w283]
              tunnel: w256 -> [w273 _]
              tunnel: w255 -> [w272 _]
              frame No Error {
                n138 = property class="Subsystem CryoCooler.lvclass"(reference=w281) -> (reference out=w278:refnum<class "Subsystem CryoCooler.lvclass">, "cmd q"=w276:T7)  [unwired: 1 in, 1 out]
                n139 = Bundle By Name(cluster=T14 {"Source"="Add Channels", "Type"="Command", "Data"=variant} ("element"), "Data"=w273) -> (w274:T14)
                n140 = call "CC System Message.vi"("Message"=w277) -> ()  [unwired: 10 in, 1 out]
                n141 = Bundle By Name(cluster=w279, "SS.CryoCooler"=w278, "Cmd Qs.Focus Q"=w276) -> (w280:T13)
                n142 = Enqueue Element(queue=w272, element=w274) -> ()  [unwired: 2 in, 3 out]
              }
              frame Error {
                n143 = Unbundle By Name(w285) -> ("source"=w284:string)
                n144 = Bundle By Name(cluster=w289, "SS.CryoCooler"=w283, "error"=w285) -> (w288:T13)
                n145 = Format Into String(format string="Error: %s", initial string=w286, w284) -> (resulting string=w282:string)  [unwired: 1 in, 1 out]
                n146 = call "CC System Message.vi"("Message"=w282) -> ()  [unwired: 10 in, 1 out]
              }
            }
          }
          frame "init pressure monitor" {
            n147 = Unbundle By Name(w305) -> ("Data Q"=w291:refnum<queue>, "SS.Pressure"=w299:refnum<class "Subsystem Pressure Monitor.lvclass">, "Hardware.Installed Hardware"=w300:T5[])
            n148 = call "CC Get Current Device.vi"("Device Type Name"="pressure monitor", "Hardware.Installed Hardware"=w300) -> ("error out"=w296:errorcluster, "Curr Device Name"=w297:string)  [unwired: 7 in, 1 out]
            n149 = call-dynamic "SS Class Init.vi"("VI Refnum"=refnum<vi> refnum, "error in (no error)"=w296, "Device"=w297, "Subsystem Pressure Monitor in"=w299) -> ("error out"=w294:errorcluster, "Channel List"=w292:refnum<class "HK Item.lvclass">[], "Subsystem Pressure Monitor out"=w295:refnum<class "Subsystem Pressure Monitor.lvclass">)  [unwired: 5 in]
            n150 = call "SS Read vi ref.vi"("error in (no error)"=w294, "Subsystem Class in"=w295) -> ("error out"=w293:errorcluster, "vi ref"=w290:refnum<vi>, "Subsystem Class out"=w302:refnum<class "Subsystem Pressure Monitor.lvclass">)  [unwired: 7 in]
            n151 = Format Into String(format string="Initializing Pressure Monitor  System %s.", w297) -> (resulting string=w303:string)  [unwired: 2 in, 1 out]
            n152 = invoke on="Pressure Panel" class="SubPnl" method="Insert VI"("VI Ref"=w290) -> ()  [unwired: 3 in, 4 out]
            n153 = case shown="No Error" w293 {
              selector: w293 -> [_ w320]
              tunnel: w303 -> [w312 w321]
              tunnel: w305 -> [w314 w324]
              tunnel: [w315 w323] -> w306
              tunnel: w302 -> [w316 w318]
              tunnel: w292 -> [w308 _]
              tunnel: w291 -> [w307 _]
              frame No Error {
                n154 = property class="Subsystem Pressure Monitor.lvcl"(reference=w316) -> (reference out=w313:refnum<class "Subsystem Pressure Monitor.lvclass">, "cmd q"=w311:T7)  [unwired: 1 in, 1 out]
                n155 = Bundle By Name(cluster=T14 {"Source"="Add Channels", "Type"="Command", "Data"=variant} ("element"), "Data"=w308) -> (w309:T14)
                n156 = call "CC System Message.vi"("Message"=w312) -> ()  [unwired: 10 in, 1 out]
                n157 = Bundle By Name(cluster=w314, "SS.Pressure"=w313, "Cmd Qs.Focus Q"=w311) -> (w315:T13)
                n158 = Enqueue Element(queue=w307, element=w309) -> ()  [unwired: 2 in, 3 out]
              }
              frame Error {
                n159 = Unbundle By Name(w320) -> ("source"=w319:string)
                n160 = Bundle By Name(cluster=w324, "SS.Pressure"=w318, "error"=w320) -> (w323:T13)
                n161 = Format Into String(format string="Error: %s", initial string=w321, w319) -> (resulting string=w317:string)  [unwired: 1 in, 1 out]
                n162 = call "CC System Message.vi"("Message"=w317) -> ()  [unwired: 10 in, 1 out]
              }
            }
          }
          frame "init scripting" {
            n163 = Unbundle By Name(w327) -> ("Cmd Qs"=w330:T6)
            n164 = vi-ref "CC Script GUI.vi"() -> (w339:refnum<vi>)
            n165 = Obtain Queue(name (unnamed)="Script Queue", element data type=T16 {"Cmd"="", "Parameters"=variant}) -> (queue out=w331:refnum<queue>)  [unwired: 3 in, 2 out]
            n166 = property class="VI (strict)"(reference=w339) -> (error out=w340:errorcluster, "Path"=w338:path)  [unwired: 1 in, 1 out]
            n167 = Bundle By Name(cluster=w330, "Script Q"=w331) -> (w329:T6)
            n168 = Open VI Reference(type specifier VI Refnum (for type only)=w339, vi path=w338, options=128, error in (no error)=w340) -> (vi reference=w337:refnum<vi>, error out=w335:errorcluster)  [unwired: 2 in]
            n169 = call-by-ref "Start Asynchronous Call"(reference=w337, error in=w335, "Standalone"=FALSE, "Cmd Qs"=w329) -> (error out=w334:errorcluster)  [unwired: 10 in, 1 out]
            n170 = Bundle By Name(cluster=w327, "Cmd Qs"=w329) -> (w328:T13)
            n171 = invoke on="Scripting Panel" class="SubPnl" method="Insert VI"(error in=w334, "VI Ref"=w339) -> (error out=w325:errorcluster)  [unwired: 2 in, 3 out]
            n172 = call <vilib>:"Clear Errors.vi"("error in (no error)"=w325) -> ()  [unwired: 5 in, 2 out]
          }
          frame "init observation list" {
            n173 = call "CC Get Filter Names.vi"() -> ("filter names"=w364:cluster{"Names":string[]}[])  [unwired: 9 in, 2 out]
            n174 = Unbundle By Name(w356) -> ("System Settings.Obs File"=w354:path, "state"=w355:refnum<user-event>)
            n175 = vi-ref "CC Observation Queue GUI.vi"() -> (w347:refnum<vi>)
            n176 = Index Array(array=w364) -> (element #1=w363:cluster{"Names":string[]}, element #2=w361:cluster{"Names":string[]})  [unwired: 2 in]
            n177 = property class="VI (strict)"(reference=w347) -> (error out=w352:errorcluster, "Path"=w351:path)  [unwired: 1 in, 1 out]
            n178 = Unbundle(w363) -> ("Names"=w362:string[])
            n179 = Unbundle(w361) -> ("Names"=w360:string[])
            n180 = property on="Filter 2" class="Ring (strict)"("Strings []"=w360) -> ()  [unwired: 2 in, 2 out]
            n181 = property on="Filter 1" class="Ring (strict)"("Strings []"=w362) -> ()  [unwired: 2 in, 2 out]
            n182 = Empty String/Path?(string/path=w354) -> (empty?=w359:bool)
            n183 = Open VI Reference(type specifier VI Refnum (for type only)=w347, vi path=w351, options=128, error in (no error)=w352) -> (vi reference=w350:refnum<vi>, error out=w348:errorcluster)  [unwired: 2 in]
            n184 = case shown="False" w359 {
              tunnel: [w371 _] -> w358
              tunnel: w355 -> [w370 _]
              tunnel: w354 -> [w367 _]
              tunnel: [w368 _] -> w345
              tunnel: [w367 _] -> w344
              tunnel: i32[] [0] ("Value (Signaling)") -> [w366 _]
              frame False {
                n185 = call "CC Rd Wr Observation List.vi"("filepath"=w367) -> ("Observation List"=w371:T9[])  [unwired: 7 in, 3 out]
                n186 = Generate User Event(user event=w370, event data cluster="show observation" ("event data")) -> (error out=w365:errorcluster)  [unwired: 2 in, 1 out]
                n187 = property on="Observation List" class="MCListbox (strict)"(error in=w365, "Val(Sgnl)"=w366) -> ()  [unwired: 1 in, 2 out]
                n188 = Strip Path(path=w367) -> (name=w368:string)  [unwired: 1 out]
              }
              frame True {
              }
            }
            "Observation File" <- w345
            n189 = call-by-ref "Start Asynchronous Call"(reference=w350, error in=w348) -> (reference out=w346:refnum<vi>)  [unwired: 12 in, 1 out]
            n190 = invoke class="VI (strict)" method="FP.Open"(reference=w346, "Activate"=TRUE ("Activate?")) -> (reference out=w343:refnum<vi>)  [unwired: 3 in, 4 out]
            n191 = call "CC create observation queue.vi"() -> ("Observation Queue"=w353:refnum<queue>)  [unwired: 10 in, 1 out]
            n192 = Bundle By Name(cluster=w356, "Queue vi ref"=w343, "Obs Queue"=w353, "Observation List"=w358, "System Settings.Obs File"=w344) -> (w357:T13)
          }
          frame "save observation" {
            n193 = Unbundle By Name(w375) -> ("Observation List"=w374:T9[], "System Settings.Obs File"=w373:path)
            n194 = Empty String/Path?(string/path=w373) -> (empty?=w372:bool)
            n195 = case shown="False" w372 {
              tunnel: w374 -> [w377 _]
              tunnel: w373 -> [w376 _]
              frame False {
                n196 = call "CC Rd Wr Observation List.vi"("filepath"=w376, "Write? (F:Read)"=TRUE, "Observation List"=w377) -> ()  [unwired: 5 in, 4 out]
              }
              frame True {
              }
            }
          }
          frame "show observation" {
            n197 = Unbundle By Name(w382) -> ("Observation List"=w381:T9[])
            n198 = call "CC Observation List to Table.vi"("Observation List"=w381) -> ("Screen Ready Table"=w379:string[][])  [unwired: 7 in, 3 out]
            n199 = call "CC Observation File Header.vi"() -> ("Header"=w380:string[])  [unwired: 10 in, 1 out]
            n200 = property on="Observation List" class="MCListbox (strict)"("ItemNames"=w379, "ColHdrString"=w380) -> ()  [unwired: 2 in, 2 out]
          }
          frame "generate script" {
            n201 = Unbundle By Name(w385) -> ("Cmd Qs.Script Q"=w388:T7, "System Settings.Obs File"=w384:path, "Observation List"=w398:T9[])
            n202 = call "Rd Wr Script Defaults.vi"() -> ("error out"=w387:errorcluster, "Script Settings"=w390:T26)  [unwired: 10 in]
            n203 = for {
              tunnel: w398 -> [w402] mode=indexing
              tunnel: [w401] -> w391 mode=concatenating
              shift-right: [w400] -> w386
              shift-left: w387 -> [w399]
              n204 = call "CC Observation to Script.vi"("error in (no error)"=w399, "Observation"=w402) -> ("error out"=w400:errorcluster, "Script Steps"=w401:T19[])  [unwired: 8 in]
            }
            n205 = call <vilib>:"Get File Extension.vi"("file"=w384) -> ("filename without extension"=w383:string)  [unwired: 6 in, 4 out]
            n206 = Unbundle By Name(w390) -> ("Script Path"=w389:path)
            n207 = call <vilib>:"Simple Error Handler.vi"("error in (no error)"=w386) -> ()  [unwired: 4 in, 5 out]
            n208 = Bundle By Name(cluster=T18 {"Name"="", "Script"=[]} ("Script"), "Name"=w383, "Script"=w391) -> (w396:T18)
            n209 = Bundle By Name(cluster=T16 {"Cmd"="", "Parameters"=variant} ("element"), "Cmd"="set script", "Parameters"=w383) -> (w393:T16)
            n210 = call "CC Rd Wr Script.vi"("Script Path"=w389, "Action"=CC_Rd_Wr_Script_Action."Write", "Script"=w396) -> ()  [unwired: 3 in, 6 out]
            n211 = Enqueue Element(queue=w388, element=w393) -> ()  [unwired: 2 in, 3 out]
          }
          frame "Check Alarms" {
            n212 = Unbundle By Name(w403) -> ("Cmd Qs.Script Q"=w405:T7, "Script Running"=w408:bool)
            n213 = call "CC Alarm Object.vi"("Alarm Action"=CC_enum_Alarm_Action."Get Alarms") -> ("Alarm List"=w420:T27[], "Alarm?"=w406:bool)  [unwired: 8 in, 1 out]
            "Alarm Status" <- w406
            n214 = And(x=w408, y=w406) -> (x .and. y?=w407:bool)
            n215 = for {
              tunnel: w420 -> [w436] mode=indexing
              tunnel: [w435] -> w419 mode=indexing
              tunnel: [w432] -> w410 mode=indexing
              n216 = Unbundle By Name(w436) -> ("Message"=w434:string, "Source"=w435:string)
              n217 = Concatenate Strings(w434, "\r\n") -> (w432:string)
            }
            n218 = case shown="True" w407 {
              tunnel: w405 -> [_ w427]
              tunnel: w403 -> [w422 w425]
              tunnel: [w422 w423] -> w404
              frame False {
              }
              frame True {
                n219 = Enqueue Element(queue=w427, element=T16 {"Cmd"="abort script", "Parameters"=variant}) -> ()  [unwired: 2 in, 3 out]
                n220 = Bundle By Name(cluster=w425, "Script Running"=FALSE) -> (w423:T13)
              }
            }
            n221 = for {
              tunnel: w419 -> [w431]
              tunnel: string[] ["Detector", "Filter Wheel", "Telescope", "Pressure Monitor", "CryoCooler", "CryoServer"] -> [w430] mode=indexing
              tunnel: [w428] -> w417 mode=indexing
              n222 = Search 1D Array(1D array=w431, element=w430) -> (index of element=w429:i32)  [unwired: 1 in]
              n223 = Greater Or Equal To 0?(x=w429) -> (x >= 0?=w428:bool)
            }
            n224 = Concatenate Strings(w410) -> (→"Alarm Message":string)
            n225 = Index Array(array=w417) -> (element #1=→"Detector Alarm":bool, element #2=→"FW Alarm":bool, element #3=→"Telescope Alarm":bool, element #4=→"Pressure Alarm":bool, element #5=→"Cryo Alarm":bool, element #6=→"Temp":bool)  [unwired: 6 in]
          }
          frame "Update Table" {
            n226 = call "Elapsed Time"() -> ("Time has Elapsed"=w445:bool)  [unwired: 12 in, 7 out]
            n227 = Unbundle By Name(w448) -> ("Data Q"=w446:refnum<queue>, "state"=w444:refnum<user-event>)
            n228 = call "CC Log Object.vi"("Action"=CC_enum_Current_Values_Action."Get Current Values") -> ("error out"=w452:errorcluster, "HK Channel out"=w443:refnum<class "HK Table.lvclass">)  [unwired: 8 in, 1 out]
            n229 = case shown="True" w445 {
              tunnel: w444 -> [_ w458]
              frame False {
              }
              frame True {
                n230 = Generate User Event(user event=w458, event data cluster="Show Plot" ("event data")) -> ()  [unwired: 2 in, 2 out]
              }
            }
            n231 = call "CC Past Noon Check.vi"() -> ("Passed noon"=w447:bool)  [unwired: 10 in, 1 out]
            n232 = call-dynamic "HK Channel Get Formatted Value Table.vi"("error in (no error)"=w452, "HK Table in"=w443) -> ("Hdr"=w450:string[], "Table"=w451:string[][])  [unwired: 5 in, 3 out]
            n233 = case shown="True" w447 {
              tunnel: w446 -> [_ w460]
              frame False {
              }
              frame True {
                n234 = Enqueue Element(queue=w460, element=T14 {"Source"="New File", "Type"="Command", "Data"=variant}) -> ()  [unwired: 2 in, 3 out]
              }
            }
            n235 = for {
              tunnel: w443 -> [w456]
              tunnel: string[] ["Telescope RA", "Telescope DEC"] -> [w455] mode=indexing
              tunnel: [w454] -> w441 mode=indexing
              tunnel: [w453] -> w437
              n236 = call-dynamic "HK Channel Read Formatted Value.vi"("Name"=w455, "HK Channel in"=w456) -> ("error out"=w453:errorcluster, "Value"=w454:dbl)  [unwired: 2 in, 6 out]
            }
            n237 = property on="Channels" class="MCListbox (strict)"("ItemNames"=w451, "ColHdrString"=w450) -> ()  [unwired: 2 in, 2 out]
            n238 = Array To Cluster(array=w441) -> (cluster=w440:cluster{"[0]":dbl, "[1]":dbl})
            n239 = call <vilib>:"Clear Errors.vi"("error in (no error)"=w437) -> ()  [unwired: 5 in, 2 out]
            n240 = call "CC Convert RA and DEC to HHMMSS.vi"("RA and DEC"=w440) -> ("DEC String"=→"Current DEC":string, "RA String"=→"Current RA":string)  [unwired: 7 in, 2 out]
          }
          frame "Show Plot" {
            n241 = property on="Channels" class="MCListbox (strict)"() -> ("ItemNames"=w473:string[][])  [unwired: 2 in, 2 out]
            n242 = for {
              tunnel: w473 -> [w502]
              tunnel: "Channels" -> [w501] mode=indexing
              tunnel: [w499] -> w469 mode=indexing
              tunnel: [w498] -> w471 mode=indexing
              n243 = Index Array(array=w502, index (row)=w501, index (col)=3 ("disabled index (col)")) -> (element=w498:string)
              n244 = Index Array(array=w502, index (row)=w501, index (col)=0 ("disabled index (col)")) -> (element=w499:string)
            }
            n245 = call "CC Read Channels from TDMS File.vi"("Sources"=w471, "ItemNames"=w469) -> ("error out"=w468:errorcluster, "units"=w462:string[], "Y Axes"=w467:i32[], "XY Graph"=w470:cluster{timestamp[], dbl[]}[])  [unwired: 6 in]
            n246 = Array Size(array=w462) -> (size(s)=w461:i32)
            n247 = for {
              N: 3 -> [_]
              tunnel: [w478] -> w464
              tunnel: w461 -> [w476]
              i -> [w477]
              n248 = Less?(x=w477, y=w476) -> (x < y?=w475:bool)
              n249 = property on="XY Graph" class="XYGraph (strict)"("ActYScl"=w477, "YScale.Visible"=w475) -> (error out=w478:errorcluster)  [unwired: 2 in, 1 out]
            }
            n250 = flat-sequence {
              tunnel: w470 -> [w482]
              tunnel: w468 -> [w481]
              tunnel: w467 -> [w480]
              tunnel: [w480] -> w466
              tunnel: w462 -> [w479]
              tunnel: [w479] -> w465
              tunnel: w464 -> [_]
              tunnel: w469 -> [w488]
              tunnel: w466 -> [w487]
              tunnel: w465 -> [w486]
              frame #0 {
                n251 = call <vilib>:"Clear Errors.vi"("error in (no error)"=w481) -> ()  [unwired: 5 in, 2 out]
                "XY Graph" <- w482
              }
              frame #1 {
                n252 = for {
                  N: 3 -> [_]
                  tunnel: w486 -> [w491] mode=indexing
                  tunnel: [w489] -> w483
                  i -> [w492]
                  n253 = property on="XY Graph" class="XYGraph (strict)"("ActYScl"=w492, "YScale.NameLbl.Text"=w491, "YScale.Visible"=TRUE ("Y Scale.Visible")) -> (error out=w489:errorcluster)  [unwired: 2 in, 1 out]
                }
                n254 = for {
                  N -> [w495]
                  tunnel: w488 -> [w496] mode=indexing
                  tunnel: w487 -> [w494] mode=indexing
                  tunnel: [w493] -> w484
                  i -> [w497]
                  n255 = property on="XY Graph" class="XYGraph (strict)"("Active Plot"=w497, "Plot.Plot Name"=w496, "LegNumRows"=w495, "Plot.YScaleIdx"=w494) -> (error out=w493:errorcluster)  [unwired: 2 in, 1 out]
                }
                n256 = call <vilib>:"Clear Errors.vi"("error in (no error)"=w484) -> ()  [unwired: 5 in, 2 out]
                n257 = call <vilib>:"Clear Errors.vi"("error in (no error)"=w483) -> ()  [unwired: 5 in, 2 out]
              }
            }
          }
          frame "Script Status" {
            n258 = Unbundle By Name(w504) -> ("Status Data"=w514:variant)
            n259 = Variant To Data(type=T23 {"Time"=timestamp(0 s since 1904-01-01), "Running"=FALSE, "Step"=0, "Script Name"="", "Step Name"=""}, Variant=w514) -> (data=w513:T23)  [unwired: 1 in, 1 out]
            n260 = Unbundle By Name(w513) -> ("Step"=w511:i32, "Step Name"=w507:string, "Running"=w506:bool)
            n261 = Format Into String(format string="Step %d: %s", w511, w507) -> (resulting string=w510:string)  [unwired: 2 in, 1 out]
            n262 = Select(t=w510, s=w506, f="Idle") -> (s? t:f=→"Status":string)
            n263 = Bundle By Name(cluster=w504, "Script Running"=w506) -> (w505:T13)
          }
          frame "New Image", "Script New Images" {
            n264 = Unbundle By Name(w518) -> ("state"=w517:refnum<user-event>)
            n265 = Generate User Event(user event=w517, event data cluster="Load Image Folder" ("event data")) -> ()  [unwired: 2 in, 2 out]
          }
          frame "Load Image Folder" {
            n266 = Unbundle By Name(w524) -> ("System Settings.Images Folder"=w522:path)
            n267 = disable-structure shown="Disabled" {
              disable-tunnel: w522 -> [w528 _]
              frame Disabled {
                n268 = control-ref of="Recent Images"() -> (w526:refnum<vi>)
                n269 = invoke on="Invoke Node" class="LstBox (strict)" method="Edit Tree Items.Delete"(reference=w526) -> (reference out=w525:refnum<vi>)  [unwired: 4 in, 4 out]
                n270 = call "CC GUI Recursive Load Folder to Tree.vi"("Tree Ref"=w525, "Depth"=3, "Path"=w528) -> ()  [unwired: 8 in, 1 out]
              }
              frame Enabled {
              }
            }
            n271 = List Folder(path=w522, pattern="*.fits") -> (filenames=w521:string[])  [unwired: 2 in, 3 out]
            n272 = call "Sort 1D Array.vim"("unsorted array"=w521) -> ("sorted array"=w520:string[])  [unwired: 10 in]
            n273 = Reverse 1D Array(array=w520) -> (reversed array=w519:string[])
            n274 = property on="Recent Images" class="LstBox (strict)"("Item Names"=w519) -> ()  [unwired: 2 in, 2 out]
          }
          frame "Load Image" {
            n275 = Unbundle By Name(w531) -> ("state"=w534:refnum<user-event>, "curr image"=w530:path)
            n276 = Generate User Event(user event=w534, event data cluster="Update Zoom" ("event data")) -> ()  [unwired: 2 in, 2 out]
            n277 = call "CC FITS Read Image.vi"("FITS File Path"=w530) -> ("Image"=w529:sgl[][])  [unwired: 9 in, 1 out]
            "Thumbnail" <- w529
            n278 = Bundle By Name(cluster=w531, "image"=w529) -> (w532:T13)
          }
          frame "Update Zoom" {
            n279 = property on="Zoom" class="IntGraph (strict)"() -> ("Plot Bounds"=w557:T28)  [unwired: 2 in, 2 out]
            n280 = property on="Thumbnail" class="IntGraph (strict)"() -> ("Cursor.Cursor Y"=w550:dbl, "Cursor.Cursor X"=w548:dbl)  [unwired: 2 in, 2 out]
            n281 = Unbundle By Name(w557) -> ("Right"=w555:i16, "Left"=w556:i16, "Bottom"=w554:i16, "Top"=w553:i16)
            n282 = Subtract(x=w555, y=w556) -> (x-y=w542:i16)
            n283 = Subtract(x=w554, y=w553) -> (x-y=w536:i16)
            n284 = Unbundle By Name(w551) -> ("image"=w549:sgl[][])
            n285 = Divide(x=w542, y=i16 2) -> (x/y=w539:dbl)
            n286 = Subtract(x=w550, y=w539) -> (x-y=w540:dbl)
            n287 = Divide(x=w536, y=i16 2) -> (x/y=w535:dbl)
            n288 = Subtract(x=w548, y=w535) -> (x-y=w538:dbl)
            n289 = Index Array(array=w549, index (col)=w548) -> (element=w546:sgl[])  [unwired: 1 in]
            n290 = Index Array(array=w549, index (row)=w550) -> (element=w547:sgl[])  [unwired: 1 in]
            n291 = Array Subset(array=w549, index (row)=w540, length (row)=w542, index (col)=w538, length (col)=w536) -> (→"Zoom":sgl[][])
            n292 = Bundle("image"=w547) -> (w545:cluster{"image":sgl[]})  [unwired: 1 in]
            n293 = Bundle("image"=w546) -> (w544:cluster{"image":sgl[]})  [unwired: 1 in]
            n294 = Build Array(w545, w544) -> (→"Waveform Graph":cluster{"image":sgl[]}[])
          }
          frame "Shutdown" {
            n295 = Unbundle By Name(w559) -> ("state"=w565:refnum<user-event>, "System Settings"=w561:T8)
            n296 = call "CC System Message.vi"("Message"="System Shutdown Starting") -> ()  [unwired: 10 in, 1 out]
            n297 = Generate User Event(user event=w565, event data cluster="shutdown subsystems" ("event data")) -> (user event out=w564:refnum<user-event>)  [unwired: 2 in, 1 out]
            n298 = call "Rd Wr System Settings.vi"("Write? (F:Read)"=TRUE, "System Settings"=w561) -> ()  [unwired: 8 in, 2 out]
            n299 = Generate User Event(user event=w564, event data cluster="shutdown all" ("event data")) -> ()  [unwired: 2 in, 2 out]
          }
          frame "shutdown subsystems" {
            n300 = Unbundle By Name(w568) -> ("SS"=w567:T29)
            n301 = Cluster To Array(cluster=w567) -> (array=w566:refnum<class "Subsystem Class.lvclass">[])
            n302 = for {
              tunnel: w566 -> [w570] mode=indexing
              n303 = call-dynamic "SS Close.vi"("Subsystem Class in"=w570) -> ("error out"=w571:errorcluster)  [unwired: 9 in, 1 out]
              n304 = call <vilib>:"Clear Errors.vi"("error in (no error)"=w571) -> ()  [unwired: 5 in, 2 out]
            }
          }
          frame "shutdown all" {
            # "Empty array to plot memory"
            n305 = Unbundle By Name(w578) -> ("Quad Viewer Ref"=w575:refnum<vi>, "Viewer Ref"=w576:refnum<vi>, "Cmd Qs.Script Q"=w580:T7, "Data Q"=w583:refnum<queue>, "Obs Queue"=w573:refnum<queue>)
            n306 = Enqueue Element(queue=w573, element=T24 {"Msg"="shutdown", "Data"=variant}) -> ()  [unwired: 2 in, 3 out]
            n307 = Build Array(w575, w576) -> (w574:refnum<vi>[])
            n308 = for {
              tunnel: w574 -> [w584] mode=indexing
              n309 = invoke class="VI" method="Abort VI"(reference=w584) -> (reference out=w586:refnum<vi>, error out=w587:errorcluster)  [unwired: 2 in, 1 out]
              n310 = Close Reference(reference=w586, error in (no error)=w587) -> (error out=w585:errorcluster)
              n311 = call <vilib>:"Clear Errors.vi"("error in (no error)"=w585) -> ()  [unwired: 5 in, 2 out]
            }
            n312 = Enqueue Element(queue=w583, element=T14 {"Source"="Shutdown", "Type"="Command", "Data"=variant}) -> ()  [unwired: 2 in, 3 out]
            n313 = Enqueue Element(queue=w580, element=T16 {"Cmd"="Shutdown", "Parameters"=variant}) -> ()  [unwired: 2 in, 3 out]
            n314 = local write "Thumbnail"(sgl[][] [] ("Thumbnail")) -> ()
          }
        }
      }
      event Menu Selection (User) {
        n315 = event-data() -> ("ItemTag"=w590:string)  [unwired: 1 in, 1 out]
        n316 = case shown="\"Restore Previous Setup\"" w590 {
          selector: w590 -> [w593 _ _ _ _]
          tunnel: w589 -> [w591 w595 w596 w608 w620]
          tunnel: [w591 w595 w596 w605 w620] -> w588
          frame "True", Default {
            n317 = Format Into String(format string="Main Menu Item %s not implemented.", w593) -> (resulting string=w592:string)  [unwired: 2 in, 1 out]
            n318 = One Button Dialog(message=w592) -> ()  [unwired: 1 in, 1 out]
          }
          frame "Edit FITS Header" {
            n319 = call "CC FITS Make FITS Header Table.vi"() -> ()  [unwired: 12 in]
          }
          frame "Restore Previous Setup" {
            n320 = Unbundle By Name(w596) -> ("state"=w598:refnum<user-event>)
            n321 = call "CC Restore Previous Setup.vi"() -> ("Select File"=w597:path, "Restored?"=w599:bool)  [unwired: 10 in]
            n322 = case shown="True" w599 {
              tunnel: w598 -> [_ w604]
              tunnel: w597 -> [_ w601]
              frame False {
              }
              frame True {
                n323 = Generate User Event(user event=w604, event data cluster="Shutdown" ("event data")) -> ()  [unwired: 2 in, 2 out]
                n324 = Format Into String(format string="User restored setup file from config archive. Restored to %s. System shutting down for restart.", w601) -> (resulting string=w600:string)  [unwired: 2 in, 1 out]
                n325 = call "CC System Message.vi"("Message"=w600) -> ()  [unwired: 10 in, 1 out]
              }
            }
          }
          frame "Select Hardware" {
            n326 = Unbundle By Name(w608) -> ("state"=w607:refnum<user-event>, "Hardware"=w611:T4)
            n327 = call "CC Hardware Config Dialog.vi"() -> ("Hardware Config"=w609:T4)  [unwired: 11 in]
            n328 = Not Equal?(x=w611, y=w609) -> (x != y?=w610:bool)
            n329 = case shown="True" w610 {
              tunnel: w609 -> [_ w616]
              tunnel: w608 -> [w612 w617]
              tunnel: w607 -> [_ w615]
              tunnel: string[] ["shutdown subsystems", "init subsystems"] -> [_ w614]
              tunnel: [w612 w613] -> w605
              frame False {
              }
              frame True {
                n330 = for {
                  tunnel: w615 -> [w619]
                  tunnel: w614 -> [w618] mode=indexing
                  n331 = Generate User Event(user event=w619, event data cluster=w618) -> ()  [unwired: 2 in, 2 out]
                }
                n332 = Bundle By Name(cluster=w617, "Hardware"=w616) -> (w613:T13)
              }
            }
          }
          frame "Exit" {
            n333 = Unbundle By Name(w620) -> ("state"=w622:refnum<user-event>)
            n334 = Generate User Event(user event=w622, event data cluster="Shutdown" ("event data")) -> ()  [unwired: 2 in, 2 out]
          }
        }
      }
      event "Observation List": Value Change {
        n335 = event-data() -> ()  [unwired: 1 in, 1 out]
        n336 = Unbundle By Name(w654) -> ("Observation List"=w653:T9[])
        n337 = Index Array(array="Observation List") -> (element=w632:i32)  [unwired: 1 in]
        n338 = Index Array(array=w653, index=w632) -> (element=w651:T9)
        n339 = Unbundle By Name(w651) -> ("Priority"=w624:i32, "ID"=w631:string, "Observer"=w650:string, "Obj Name"=w649:string, "RA and DEC String.RA"=w648:string, "RA and DEC String.DEC"=w647:string, "Filter Wheel 1"=w645:string, "Filter Wheel 2"=w637:string, "Dither Options.Dither"=w636:T2, "Dither Options.Dither Radius"=w635:dbl, "Integration Time"=w634:dbl, "Dither Options.Dither Points"=w633:i32, "Obj Type"=w630:string, "Images"=w629:i32, "Dither Options.Dither Phase"=w628:dbl, "Offsets.RA"=w627:dbl, "Offsets.DEC"=w626:dbl, "Offsets.ROT"=w625:dbl, "Comment 1"=w623:string)
        n340 = local write "Obj Name"(w649) -> ()
        n341 = local write "Observer"(w650) -> ()
        n342 = local write "Block ID"(w631) -> ()
        n343 = local write "Priority"(w624) -> ()
        n344 = local write "DEC"(w647) -> ()
        n345 = local write "RA"(w648) -> ()
        n346 = local write "ROT Offset"(w625) -> ()
        n347 = local write "Comment"(w623) -> ()
        n348 = local write "DECoffset"(w626) -> ()
        n349 = local write "Obj Type"(w630) -> ()
        n350 = local write "RAoffset"(w627) -> ()
        n351 = local write "Int Time"(w634) -> ()
        n352 = local write "Images"(w629) -> ()
        n353 = local write "Radius"(w635) -> ()
        n354 = local write "Dither"(w636) -> ()
        n355 = local write "Phase"(w628) -> ()
        n356 = local write "Spots"(w633) -> ()
        n357 = property on="Filter 1" class="Ring (strict)"() -> ("Strings []"=w646:string[])  [unwired: 2 in, 2 out]
        n358 = property on="Filter 2" class="Ring (strict)"() -> ("Strings []"=w639:string[])  [unwired: 2 in, 2 out]
        n359 = Search 1D Array(1D array=w639, element=w637) -> (index of element=w640:i32)  [unwired: 1 in]
        n360 = Search 1D Array(1D array=w646, element=w645) -> (index of element=w644:i32)  [unwired: 1 in]
        n361 = Max & Min(x=w640, y=0) -> (max(x,y)=w638:i32)  [unwired: 1 out]
        n362 = Max & Min(x=w644, y=0) -> (max(x,y)=w642:i32)  [unwired: 1 out]
        n363 = property on="Filter 2" class="Ring (strict)"("Value"=w638) -> ()  [unwired: 2 in, 2 out]
        n364 = property on="Filter 1" class="Ring (strict)"("Value"=w642) -> ()  [unwired: 2 in, 2 out]
      }
      event "Observation List": Shortcut Menu Activation? {
        n365 = event-data() -> ()  [unwired: 1 in, 7 out]
        n366 = event-data("Discard?"=FALSE) -> ()  [unwired: 1 in, 1 out]
      }
      event "Observation List": Shortcut Menu Selection (User) {
        n367 = event-data() -> ("ItemTag"=w664:string, "CtlRef"=w666:refnum<vi>, "Coords"=w665:T30)  [unwired: 1 in]
        n368 = invoke class="MCListbox (strict)" method="Point To Row Column"(reference=w666, "Point"=w665) -> ("CellPosition"=w662:T31)  [unwired: 5 in, 6 out]
        n369 = Unbundle By Name(w659) -> ("Observation List"=w663:T9[])
        n370 = Unbundle By Name(w659) -> ("state"=w658:refnum<user-event>)
        n371 = case shown="\"Delete Item\"" w664 {
          tunnel: w663 -> [w667 w671]
          tunnel: w662 -> [_ w670]
          tunnel: [w667 w668] -> w660
          frame "False", Default {
          }
          frame "Delete Item" {
            n372 = Unbundle By Name(w670) -> ("Row"=w669:i32)
            n373 = Delete From Array(array=w671, index=w669) -> (array with subset deleted=w668:T9[])  [unwired: 1 in, 1 out]
          }
        }
        n374 = Generate User Event(user event=w658, event data cluster="show observation" ("event data")) -> ()  [unwired: 2 in, 2 out]
        n375 = Bundle By Name(cluster=w659, "Observation List"=w660) -> (w661:T13)
      }
      event "Add to Q", "Add to Q top": Value Change {
        n376 = event-data() -> ()  [unwired: 1 in, 6 out]
        n377 = Unbundle By Name(w677) -> ("Obs Queue"=w674:refnum<queue>, "Observation List"=w676:T9[])
        n378 = local read "Observation List"() -> (w675:i32[])
        n379 = for {
          tunnel: w676 -> [w692]
          tunnel: w675 -> [w691] mode=indexing
          tunnel: w674 -> [w690]
          tunnel: "Add to Q" -> [w688]
          tunnel: CC_enum_Observation_Status."Ready" ("Observation Status") -> [w678]
          n380 = Index Array(array=w692, index=w691) -> (element=w681:T9)
          n381 = Bundle By Name(cluster=w681, "Observation Status"=w678) -> (w679:T9)
          n382 = Select(t=T24 {"Msg"="addend", "Data"=variant} ("element"), s=w688, f=T24 {"Msg"="addtop", "Data"=variant} ("element")) -> (s? t:f=w683:T24)
          n383 = Bundle By Name(cluster=w683, "Data"=w681) -> (w689:T24)
          n384 = Unbundle By Name(w679) -> ("ID"=w680:string)
          n385 = Unbundle By Name(w683) -> ("Msg"=w682:string)
          n386 = Enqueue Element(queue=w690, element=w689) -> ()  [unwired: 2 in, 3 out]
          n387 = Format Into String(format string="Sending observation %s to queue with command %s. ", w680, w682) -> (resulting string=w685:string)  [unwired: 2 in, 1 out]
          n388 = call "CC System Message.vi"("Message"=w685) -> ()  [unwired: 10 in, 1 out]
        }
      }
      event "Generate Script": Value Change {
        n389 = event-data() -> ()  [unwired: 1 in, 6 out]
        n390 = Unbundle By Name(w708) -> ("Cmd Qs.Script Q"=w696:T7, "System Settings.Obs File"=w695:path, "Observation List"=w707:T9[])
        n391 = call "Rd Wr Script Defaults.vi"() -> ("error out"=w694:errorcluster, "Script Settings"=w698:T26)  [unwired: 10 in]
        n392 = for {
          tunnel: w707 -> [w712] mode=indexing
          tunnel: [w711] -> w699 mode=concatenating
          shift-right: [w710] -> w693
          shift-left: w694 -> [w709]
          n393 = call "CC Observation to Script.vi"("error in (no error)"=w709, "Observation"=w712) -> ("error out"=w710:errorcluster, "Script Steps"=w711:T19[])  [unwired: 8 in]
        }
        n394 = Unbundle By Name(w698) -> ("Script Path"=w697:path)
        n395 = Strip Path(path=w695) -> (name=w700:string)  [unwired: 1 out]
        n396 = call <vilib>:"Simple Error Handler.vi"("error in (no error)"=w693) -> ()  [unwired: 4 in, 5 out]
        n397 = Bundle By Name(cluster=T18 {"Name"="", "Script"=[]} ("Script"), "Name"=w700, "Script"=w699) -> (w705:T18)
        n398 = Bundle By Name(cluster=T16 {"Cmd"="", "Parameters"=variant} ("element"), "Cmd"="set script", "Parameters"=w700) -> (w702:T16)
        n399 = call "CC Rd Wr Script.vi"("Script Path"=w697, "Action"=CC_Rd_Wr_Script_Action."Write", "Script"=w705) -> ()  [unwired: 3 in, 6 out]
        n400 = Enqueue Element(queue=w696, element=w702) -> ()  [unwired: 2 in, 3 out]
      }
      event "Load Obs List": Value Change {
        n401 = event-data() -> ()  [unwired: 1 in, 6 out]
        n402 = call "CC Rd Wr Observation List.vi"() -> ("file"=w715:path, "Observation List"=w716:T9[])  [unwired: 8 in, 2 out]
        n403 = Unbundle By Name(w717) -> ("state"=w713:refnum<user-event>)
        n404 = Empty Array?(array=w716) -> (empty?=w718:bool)
        n405 = case shown="False" w718 {
          tunnel: w717 -> [w724 w725]
          tunnel: w716 -> [w723 _]
          tunnel: w715 -> [w722 _]
          tunnel: [w721 w725] -> w714
          tunnel: w713 -> [w720 _]
          frame False {
            n406 = Bundle By Name(cluster=w724, "Observation List"=w723, "System Settings.Obs File"=w722) -> (w721:T13)
            n407 = Generate User Event(user event=w720, event data cluster="show observation" ("event data")) -> ()  [unwired: 2 in, 2 out]
          }
          frame True {
          }
        }
      }
      event "Save Obs List": Value Change {
        n408 = event-data() -> ()  [unwired: 1 in, 6 out]
        n409 = Unbundle By Name(w726) -> ("System Settings.Obs File"=w734:path)
        n410 = Strip Path(path=w734) -> (stripped path=w732:path, name=w733:string)
        n411 = call "File Dialog"("start path"=w732, "default name"=w733, "pattern (all files)"="*.csv") -> ("selected path"=w729:path, "cancelled"=w730:bool)  [unwired: 9 in, 2 out]
        n412 = Unbundle By Name(w726) -> ("Observation List"=w728:T9[])
        n413 = case shown="False" w730 {
          tunnel: w729 -> [w736 _]
          tunnel: w728 -> [w739 _]
          tunnel: w726 -> [w737 w740]
          tunnel: [w735 w740] -> w727
          frame False {
            n414 = call "CC Rd Wr Observation List.vi"("filepath"=w736, "Write? (F:Read)"=TRUE, "Observation List"=w739) -> ()  [unwired: 5 in, 4 out]
            n415 = Bundle By Name(cluster=w737, "System Settings.Obs File"=w736) -> (w735:T13)
          }
          frame True {
          }
        }
      }
      event "Add Obs Row", "Replace": Value Change {
        n416 = event-data() -> ("CtlRef"=w767:refnum<vi>)  [unwired: 1 in]
        n417 = property class="Bool"(reference=w767) -> ("Label.Text"=w766:string)  [unwired: 1 in, 2 out]
        n418 = property on="Filter 1" class="Ring (strict)"() -> ("Strings []"=w776:string[])  [unwired: 2 in, 2 out]
        n419 = Equal?(x=w766, y="Replace") -> (x = y?=w764:bool)
        n420 = property on="Filter 2" class="Ring (strict)"() -> ("Strings []"=w773:string[])  [unwired: 2 in, 2 out]
        n421 = Unbundle By Name(w759) -> ("state"=w758:refnum<user-event>, "Observation List"=w744:T9[])
        n422 = Index Array(array=w776, index="Filter 1") -> (element=w774:string)
        n423 = Index Array(array=w773, index="Filter 2") -> (element=w771:string)
        n424 = call "CC Observation Check For BlockID.vi"("Generate ID?"=TRUE, "BlockID"="Block ID", "Observation List"=w744) -> ("BlockID string"=w742:string)  [unwired: 6 in, 2 out]
        n425 = Generate User Event(user event=w758, event data cluster="show observation" ("event data")) -> (user event out=w748:refnum<user-event>)  [unwired: 2 in, 1 out]
        n426 = local read "Observation List"() -> (w762:i32[])
        n427 = Bundle By Name(cluster=T9 {"Priority"=0, "ID"="", "Observer"="", "Obj Name"="", "Obj Type"="", "RA and DEC String"={"RA"="12:34:56.789", "DEC"="010:11:12.013"}, "Filter Wheel 1"="", "Filter Wheel 2"="", "Integration Time"=0.0, "Observation Status"=enum."Ready", "Offsets"={"RA"=0.0, "DEC"=0.0, "ROT"=0.0}, "Images"=0, "Dither Options"={"Dither"=enum."None", "Dither Radius"=0.0, "Dither Points"=0, "Dither Phase"=0.0}, "Comment 1"="", "Comment 2"=""} ("Observation"), "ID"=w742, "Observer"="Observer", "Obj Type"="Obj Type", "Obj Name"="Obj Name", "RA and DEC String.RA"="RA", "RA and DEC String.DEC"="DEC", "Filter Wheel 1"=w774, "Filter Wheel 2"=w771, "Offsets.RA"="RAoffset", "Offsets.DEC"="DECoffset", "Offsets.ROT"="ROT Offset", "Dither Options.Dither"="Dither", "Dither Options.Dither Phase"="Phase", "Dither Options.Dither Radius"="Radius", "Integration Time"="Int Time", "Dither Options.Dither Points"="Spots", "Images"="Images", "Priority"="Priority", "Comment 1"="Comment") -> (w763:T9)
        n428 = Generate User Event(user event=w748, event data cluster="save observation" ("event data")) -> ()  [unwired: 2 in, 2 out]
        n429 = Index Array(array=w762) -> (element=w755:i32)  [unwired: 1 in]
        n430 = case shown="True" w764 {
          tunnel: w744 -> [w786 w790]
          tunnel: w763 -> [w784 w789]
          tunnel: w755 -> [_ w788]
          tunnel: [w785 w787] -> w761
          frame False {
            n431 = call "CC Next ID.vi"() -> ("BlockID string"=w782:string)  [unwired: 9 in, 2 out]
            n432 = Bundle By Name(cluster=w784, "ID"=w782) -> (w783:T9)
            n433 = Build Array (concatenate)(w786, w783) -> (w785:T9[])
          }
          frame True {
            n434 = Replace Array Subset(array=w790, new element=w789, index=w788) -> (w787:T9[])
          }
        }
        n435 = Bundle By Name(cluster=w759, "Observation List"=w761) -> (w760:T13)
      }
      event Value Change {
        n436 = event-data() -> ("NewVal"=w792:T2)  [unwired: 1 in, 5 out]
        n437 = case shown="\"None\"" w792 {
          tunnel: [T25."Disabled and Grayed Out" ("Disabled") T25."Enabled" ("Disabled")] -> w791
          frame "None" {
            n438 = property on="Spots" class="DigNum (strict)"("Value"=1 ("Spots")) -> ()  [unwired: 2 in, 2 out]
          }
          frame "Circle", Default {
          }
        }
        n439 = property on="Spots" class="DigNum (strict)"("DisabledEnum"=w791) -> ()  [unwired: 2 in, 2 out]
      }
      event "RA": Value Change {
        n440 = event-data() -> ("NewVal"=w798:string)  [unwired: 1 in, 5 out]
        n441 = call "CC Parse Right Ascension.vi"("Right Ascension string"=w798) -> ("error out"=w797:errorcluster)  [unwired: 8 in, 2 out]
        n442 = case shown="Error .." w797 {
          selector: w797 -> [_ w801]
          frame No Error {
          }
          frame Error {
            n443 = Unbundle By Name(w801) -> ("source"=w800:string)
            n444 = One Button Dialog(message=w800) -> ()  [unwired: 1 in, 1 out]
          }
        }
      }
      event "DEC": Value Change {
        n445 = event-data() -> ("NewVal"=w803:string)  [unwired: 1 in]
        n446 = call "CC Parse Declination.vi"("Declination string"=w803) -> ("error out"=w802:errorcluster)  [unwired: 8 in, 2 out]
        n447 = case shown="Error .." w802 {
          selector: w802 -> [_ w806]
          frame No Error {
          }
          frame Error {
            n448 = Unbundle By Name(w806) -> ("source"=w805:string)
            n449 = One Button Dialog(message=w805) -> ()  [unwired: 1 in, 1 out]
          }
        }
      }
      event "Log", "Log 2": Value Change {
        n450 = event-data() -> ()  [unwired: 1 in, 6 out]
        n451 = Build Array("Log", "Log 2") -> (w807:bool[])
        n452 = for {
          tunnel: w807 -> [w812] mode=indexing
          i -> [w813]
          n453 = Boolean To (0,1)(Boolean=w812) -> (0, 1=w811:i16)
          n454 = property on="XY Graph" class="XYGraph (strict)"("ActYScl"=w813, "YScale.Mapping Mode"=w811) -> ()  [unwired: 2 in, 2 out]
        }
      }
      event "XY Graph": Mouse Enter {
        n455 = event-data() -> ("CtlRef"=w815:refnum<vi>)  [unwired: 1 in]
        n456 = property class="XYGraph (strict)"(reference=w815, "Legend Visible"=TRUE ("Legend:Visible")) -> ()  [unwired: 1 in, 2 out]
      }
      event "XY Graph": Mouse Leave {
        n457 = event-data() -> ("CtlRef"=w818:refnum<vi>)  [unwired: 1 in]
        n458 = property class="XYGraph (strict)"(reference=w818, "Legend Visible"=FALSE ("Legend:Visible")) -> ()  [unwired: 1 in, 2 out]
      }
      event "Channels": Value Change {
        n459 = event-data() -> ()  [unwired: 1 in, 6 out]
        n460 = Unbundle By Name(w821) -> ("state"=w820:refnum<user-event>)
        n461 = Generate User Event(user event=w820, event data cluster="Show Plot" ("event data")) -> ()  [unwired: 2 in, 2 out]
      }
      event "Recent Images": Value Change {
        n462 = event-data() -> ("CtlRef"=w827:refnum<vi>, "NewVal"=w825:i32)  [unwired: 1 in, 1 out]
        n463 = Unbundle By Name(w828) -> ("state"=w831:refnum<user-event>, "System Settings.Images Folder"=w823:path)
        n464 = property class="LstBox (strict)"(reference=w827) -> ("Item Names"=w826:string[])  [unwired: 1 in, 2 out]
        n465 = Index Array(array=w826, index=w825) -> (element=w824:string)
        n466 = xnode "Match Regular Expression"("input string"=w824, "regular expression"="(.*\\.fits)") -> ("submatch 1"=w830:string)  [unwired: 4 in, 5 out]
        n467 = Empty String/Path?(string/path=w830) -> (empty?=w832:bool)
        n468 = case shown="False" w832 {
          tunnel: w831 -> [w840 _]
          tunnel: w830 -> [w836 _]
          tunnel: w828 -> [w838 w841]
          tunnel: [w837 w841] -> w829
          tunnel: w823 -> [w835 _]
          frame False {
            n469 = Build Path(base path=w835, name or relative path=w836) -> (appended path=w834:path)
            n470 = Generate User Event(user event=w840, event data cluster="Load Image" ("event data")) -> ()  [unwired: 2 in, 2 out]
            n471 = Bundle By Name(cluster=w838, "curr image"=w834) -> (w837:T13)
            "Current File" <- w836
          }
          frame True {
          }
        }
      }
      event "Recent Images": Shortcut Menu Activation? {
        n472 = event-data() -> ("MenuRef"=w969:refnum<k9>, "CtlRef"=w963:refnum<vi>, "Coords"=w962:T30)  [unwired: 1 in]
        n473 = property class="LstBox (strict)" props=["Item Names", "Value"](reference=w963) -> ("Item Names"=w968:string[])  [unwired: 1 in, 3 out]
        n474 = invoke class="LstBox (strict)" method="Point To Row"(reference=w963, "Point"=w962) -> ("Row"=w961:i32)  [unwired: 5 in, 6 out]
        n475 = Unbundle By Name(w966) -> ("System Settings.Images Folder"=w965:path)
        n476 = Index Array(array=w968, index=w961) -> (element=w967:string)
        n477 = Build Path(base path=w965, name or relative path=w967) -> (appended path=w964:path)
        n478 = call <vilib>:"Check if File or Folder Exists.vi"("path"=w964) -> ("file or folder exists?"=w971:bool)  [unwired: 8 in, 2 out]
        n479 = Set Menu Item Info(7:"Explore..." ("item tag"), 9:w971, 10:w967, 11:w969) -> ()  [unwired: 3 in, 2 out]
        n480 = event-data("Discard?"=FALSE) -> ()  [unwired: 1 in, 1 out]
      }
      event "Recent Images": Shortcut Menu Selection (User) {
        n481 = event-data() -> ("ItemTag"=w982:string, "CtlRef"=w975:refnum<vi>, "Coords"=w974:T30)  [unwired: 1 in]
        n482 = Unbundle By Name(w979) -> ("System Settings.Images Folder"=w977:path)
        n483 = property class="LstBox (strict)"(reference=w975) -> ("Item Names"=w980:string[])  [unwired: 1 in, 2 out]
        n484 = invoke class="LstBox (strict)" method="Point To Row"(reference=w975, "Point"=w974) -> ("Row"=w973:i32)  [unwired: 5 in, 6 out]
        n485 = Index Array(array=w980, index=w973) -> (element=w978:string)
        n486 = Build Path(base path=w977, name or relative path=w978) -> (appended path=w976:path)
        n487 = case shown="\"Open in Quad Viewer\"" w982 {
          tunnel: w979 -> [w983 w985 w992]
          tunnel: [w983 w985 w990] -> w981
          tunnel: w976 -> [_ w984 w989]
          frame "False", Default {
          }
          frame "Explore..." {
            n488 = call <vilib>:"Check if File or Folder Exists.vi"("path"=w984) -> ("file or folder exists?"=w987:bool, "dup path"=w986:path)  [unwired: 8 in, 1 out]
            n489 = case shown="True" w987 {
              tunnel: w986 -> [_ w988]
              frame False {
              }
              frame True {
                n490 = call <vilib>:"Show in File System.vi"("file or directory path"=w988) -> ()  [unwired: 10 in, 1 out]
              }
            }
          }
          frame "Open in Quad Viewer" {
            # "Add quad viwer"
            n491 = call "CC Get All Files for Image.vi"("path"=w989) -> ("Files for image"=w993:path[])  [unwired: 9 in, 1 out]
            n492 = call "CC Launch Quad Viewer.vi"("Files"=w993) -> ("reference out"=w991:refnum<vi>)  [unwired: 9 in, 1 out]
            n493 = Bundle By Name(cluster=w992, "Quad Viewer Ref"=w991) -> (w990:T13)
          }
        }
      }
      event "Thumbnail": Cursor Move {
        n494 = event-data() -> ()  [unwired: 1 in, 9 out]
        n495 = Unbundle By Name(w996) -> ("state"=w995:refnum<user-event>)
        n496 = Generate User Event(user event=w995, event data cluster="Update Zoom" ("event data")) -> ()  [unwired: 2 in, 2 out]
      }
      event "Waveform Graph": Mouse Enter {
        n497 = event-data() -> ("CtlRef"=w998:refnum<vi>)  [unwired: 1 in]
        n498 = property class="WFGraph (strict)"(reference=w998, "Legend Visible"=TRUE ("Legend:Visible")) -> ()  [unwired: 1 in, 2 out]
      }
      event "Waveform Graph": Mouse Leave {
        n499 = event-data() -> ("CtlRef"=w1000:refnum<vi>)  [unwired: 1 in]
        n500 = property class="WFGraph (strict)"(reference=w1000, "Legend Visible"=FALSE ("Legend:Visible")) -> ()  [unwired: 1 in, 2 out]
      }
      event "Send": Value Change {
        n501 = event-data() -> ()  [unwired: 1 in, 6 out]
        n502 = call "CC System Message.vi"("Message"="Note for Log") -> ()  [unwired: 10 in, 1 out]
      }
      event "Close": Value Change; Panel Close {
        n503 = event-data() -> ()  [unwired: 1 in, 3 out]
        n504 = Unbundle By Name(w1008) -> ("state"=w1007:refnum<user-event>)
        n505 = Generate User Event(user event=w1007, event data cluster="Shutdown" ("event data")) -> ()  [unwired: 2 in, 2 out]
      }
      event "Tab Control": Value Change {
        n506 = event-data() -> ()  [unwired: 1 in, 6 out]
      }
      event "Open Log": Value Change {
        n507 = event-data() -> ()  [unwired: 1 in, 1 out]
        n508 = Unbundle By Name(w1017) -> ("file path"=w1016:path, "Viewer Ref"=w1010:refnum<vi>)
        n509 = Not A Number/Path/Refnum?(number/path/refnum=w1010) -> (NaN/Path/Refnum?=w1011:bool)
        n510 = Empty String/Path?(string/path=w1016) -> (empty?=w1015:bool)
        n511 = call "CC Log Object.vi"("Action"=CC_enum_Current_Values_Action."Get Current Values") -> ("Current File"=w1014:path)  [unwired: 8 in, 2 out]
        n512 = Select(t=w1014, s=w1015, f=w1016) -> (s? t:f=w1012:path)
        n513 = case shown="True" w1011 {
          tunnel: w1017 -> [w1019 w1030]
          tunnel: [w1019 w1029] -> w1013
          tunnel: w1012 -> [_ w1023]
          tunnel: w1010 -> [w1021 _]
          frame False {
            n514 = property class="VI Interface Type 3"(reference=w1021, "Front Panel.IsFrontmost"=TRUE ("Front Panel Window:Is Frontmost")) -> ()  [unwired: 1 in, 2 out]
          }
          frame True {
            n515 = vi-ref "NI_TDMS File Viewer.lvlib:TDMS - File Viewer (NXG Style).vi"() -> (w1028:refnum<vi>)
            n516 = property class="VI Interface Type 3"(reference=w1028) -> (reference out=w1025:refnum<vi>, "Path"=w1027:path)  [unwired: 1 in, 1 out]
            n517 = Open VI Reference(type specifier VI Refnum (for type only)=w1025, vi path=w1027, options=128) -> (vi reference=w1024:refnum<vi>)  [unwired: 3 in, 1 out]
            n518 = call-by-ref "Start Asynchronous Call"(reference=w1024, "file in"=w1023) -> (reference out=w1022:refnum<vi>)  [unwired: 10 in, 3 out]
            n519 = Bundle By Name(cluster=w1030, "Viewer Ref"=w1022) -> (w1029:T13)
          }
        }
      }
      event "Edit FITS Hdr": Value Change {
        n520 = event-data() -> ()  [unwired: 1 in, 6 out]
        n521 = call "CC FITS Make FITS Header Table.vi"() -> ()  [unwired: 12 in]
      }
      event "Data Folder": Value Change {
        n522 = event-data() -> ()  [unwired: 1 in, 6 out]
        n523 = Unbundle By Name(w1037) -> ("state"=w1036:refnum<user-event>)
        n524 = Bundle By Name(cluster=w1037, "System Settings.Images Folder"="Data Folder") -> (w1034:T13)
        n525 = Generate User Event(user event=w1036, event data cluster="Load Image Folder" ("event data")) -> ()  [unwired: 2 in, 2 out]
        n526 = Unbundle By Name(w1034) -> ("System Settings"=w1033:T8)
        n527 = call "Rd Wr System Settings.vi"("Write? (F:Read)"=TRUE, "System Settings"=w1033) -> ()  [unwired: 8 in, 2 out]
      }
    }
  }
  n528 = Unbundle By Name(w7) -> ("Application:Kind"=w4:T3)
  n529 = Not Equal?(x=T3."Evaluation" ("y"), y=w4) -> (x != y?=w1:bool)
  n530 = Not Equal?(x=w4, y=T3."Development System") -> (x != y?=w5:bool)
  n531 = And(x=w1, y=w5) -> (x .and. y?=w2:bool)
  n532 = Quit LabVIEW(quit? (T)=w2) -> ()
